vi "VP_NanoPositioner_FPGA_MultiTraj.vi"() -> ()   [LabVIEW 2015]
uses:
  FPGA states.ctl
  FPGA Commands.ctl
  RT VIs/Scan type.ctl
  Data Save Trigger.ctl
  Scan Geometry.ctl
  spiral radial direction.ctl
  spiral rotation direction.ctl
  Inner Scan axis.ctl
  Scan Type and Geometry.ctl
  Data Save Flag.ctl
  <vilib>/Platform/TimedLoop/XDataNode/timing_clust.ctl
  <vilib>/Platform/TimedLoop/XDataNode/nitl_modes.ctl
  <vilib>/Platform/TimedLoop/XDataNode/wakeup.ctl
  Trajectory FGV states.ctl
  <vilib>/rvi/Emulation/niFpgaGetClockAttributes.vi
  <vilib>/rvi/Emulation/niFpgaSctlEmulationGetInTimedLoop.vi
  <vilib>/rvi/Emulation/niFpgaEmulationReportErrorSimple.vi
  <vilib>/rvi/Emulation/niFpgaEmulationIsFPGAContextNoSignature.vi
  <vilib>/rvi/DataTransferAndStorage/Container/Common/niFpgaContainerGetUniqueNameForEmu.vi
  <vilib>/rvi/Memory/Memory_Emulation/niFpgaMemoryEmulationCacheClearOnFirstRun.vi
  <vilib>/rvi/Memory/Memory_Emulation/nirvimemoryEmulationManagerCache_MakeExclusive.vi
  <vilib>/rvi/Memory/Memory_Emulation/niFpgaMemoryEmulationValidateCache.vi
  <vilib>/rvi/Memory/Memory_Emulation/nirvimemoryEmulationManagerCache_InsertValue.vi
  <vilib>/Utility/error.llb/Clear Errors.vi
  <vilib>/rvi/Memory/Memory_Emulation/nirvimemoryEmulationManagerCache_ReleaseExclusive.vi
  <vilib>/rvi/Memory/Memory_Emulation/nirvimemoryEmulationManagerCache_GetValue.vi
  <vilib>/rvi/Memory/Memory_Emulation/nirvimemoryEmulationManagerCache_SetValue.vi
  <vilib>/rvi/Emulation/niFpgaProcessEmulError.vi
  <vilib>/rvi/Emulation/niFpgaCriticalErrorInLSC.vi
  <vilib>/rvi/interface/RandomDataEmulation/niFpgaRandomDataHandleErrors.vi
  <vilib>/rvi/eio/common/nirviEmuTemplateMethod_errors.vi
  <vilib>/rvi/DataTransferAndStorage/Container/XNode/niFpgaContainer.xnode
  <vilib>/rvi/DataTransferAndStorage/Register/Emulation/niFpgaRegisterEmulation.vi
  <vilib>/rvi/interface/RandomDataEmulation/nirviRandomDataFpgaReadWriteTemplate.vi
  <vilib>/eio/EIONode/EIONode.xnode
  <vilib>/Platform/TimedLoop/XDataNode/XDataNode.xnode
  <vilib>/Platform/TimedLoop/XDataNode/XDNodeRunTimeDep.lvlib
panel:
  in  "Data Save Flag":T1=enum."Save Data"
  out "Position Number":u32
  out "Scan Type and Geometry":T2
  out "Outer Loop iterations":i32
  out "Counter Loop iterations":i32
  in  "Y Reference DC Offset (nm)":fxp<+/-,16,16>
  in  "Y Reference Amplitude (nm)":fxp<+/-,40,17>
  in  "X Reference DC Offset (nm)":fxp<+/-,16,16>
  in  "X Reference Amplitude (nm)":fxp<+/-,40,17>
  out "Controller loop iterations":i32
  out "Trajectory Complete":bool
  in  "Inner Scan axis":T3
  in  "Spiral Rotation Direction":T4
  in  "Radial direction":T5=enum."Inward"
  in  "Det Frequency":fxp<+,32,0>=0.9999999997671694
  in  "Traj Frequency":fxp<+,32,0>=0.9999999997671694
  in  "Max radius":fxp<+/-,32,16>
  in  "Spiral Step Size":fxp<+/-,32,16>
  in  "Y Step Size":fxp<+/-,24,16>
  in  "X Step Size":fxp<+/-,24,16>
  in  "Scan Geometry":T6
  out "Z Reference Loop iterations":i32
  out "XY Reference Loop iterations":i32
  in  "Data Save Trigger Source":T7
  out "FIFO loop iterations":i32
  out "Trigger Generation Loop iterations":i32
  out "Module output loop iterations":i32
  out "Plant output loop iterations":i32
  in  "Scan type":T8
  out "Interferometer Loop Error":errorcluster
  out "Wait error":errorcluster
  out "Shutdown error":errorcluster
  out "FPGA error monitor":errorcluster
  out "Run Loop error":errorcluster
  in  "Wait timer (ms)":u16=50 caption="Count(mSec)"
  in  "New FPGA command":bool
  in  "FPGA command":T9
  out "FPGA state":T10
  out "End Run Error":errorcluster
  in  "Y End (nm)":fxp<+/-,16,16>
  in  "Y Start (nm)":fxp<+/-,16,16>
  in  "X End (nm)":fxp<+/-,16,16>
  in  "X Start (nm)":fxp<+/-,16,16>
  in  "DT Reset":bool
  in  "DT Duty Cycle (periods)":fxp<+,32,0>=0.5 caption="DT duty cycle (periods)"
  in  "DT Reference DC Offset (V)":fxp<+/-,16,16>
  in  "DT Reference Amplitude (V)":fxp<+/-,40,17>
  in  "DT Phase Offset (periods)":fxp<+,32,0>
  out "Measured Z Reference Loop Period (ticks)":u32
  in  "Z Reference Loop Period (us)":u32 caption="Z Reference Time Period (uSec)"
  in  "Z Reference DC Offset (nm)":fxp<+/-,16,16>
  in  "Z Reference Amplitude (nm)":fxp<+/-,40,17>
  in  "Detector Trigger Lower Limit (V)":fxp<+/-,20,5>=-5.0
  out "Detector Trigger In Range?":bool
  in  "Detector Trigger Upper Limit (V)":fxp<+/-,20,5>=5.0
  out "Measured Trigger Generation Loop Period (Ticks)":u32
  in  "Trigger Generation Time Period (uSec)":u32
  in  "Z-Stage Scaling Direction":fxp<+/-,3,3>=-1.0
  in  "Y-Stage Scaling Direction":fxp<+/-,3,3>=-1.0
  in  "Optics and or Sample Stage":T11(ring)
  in  "Sample Z Stage Resolution (nm)":fxp<+,33,3>=0.001000046730041504
  in  "Sample Y Stage Resolution (nm)":fxp<+,33,3>=0.001000046730041504
  in  "Sample X Stage Resolution (nm)":fxp<+,33,3>=0.001000046730041504
  out "Sample Z Stage Displacement raw (nm)":fxp<+/-,32,16> format="%.62g"
  out "Sample Y Stage Displacement raw (nm)":fxp<+/-,32,16> format="%.41g"
  out "Sample X Stage Displacement raw (nm)":fxp<+/-,32,16> format="%.62g"
  in  "Reset Sample Z":bool
  in  "Reset Sample Y":bool
  in  "Reset Sample X":bool
  out "Mod6/DIO3":bool
  out "Mod6/DIO2":bool
  out "Mod5/DIO3":bool
  out "Mod5/DIO2":bool
  out "Mod4/DIO3":bool
  out "Mod4/DIO2":bool
  in  "X-Stage Scaling Direction":fxp<+/-,3,3>=-1.0
  in  "Z-Stage nm to V Scaling":fxp<+/-,32,12>
  in  "Y-Stage nm to V Scaling":fxp<+/-,32,12>
  in  "X-Stage nm to V Scaling":fxp<+/-,32,12>
  out "Kxx Output, Kxx*ex (V)":fxp<+/-,58,25>
  out "Kyy Output, Kyy*ey (V)":fxp<+/-,58,25>
  out "Kzz Output, Kzz*ez (V)":fxp<+/-,58,25>
  in  "sos gain SF Controller xx1":fxp<+/-,42,9>
  in  "-a01(2) xx1":fxp<+/-,64,9>[](array[numeric])=[0.0, 0.0, 0.0, 0.0, 0.0, 0.0, 0.0, 0.0, 0.0, 0.0, 0.0, 0.0, 0.0, 0.0, 0.0, 0.0, 0.0, 0.0, 0.0, 0.0]
  in  "-a02(2) xx1":fxp<+/-,64,9>[](array[numeric])=[0.0, 0.0, 0.0, 0.0, 0.0, 0.0, 0.0, 0.0, 0.0, 0.0, 0.0, 0.0, 0.0, 0.0, 0.0, 0.0, 0.0, 0.0, 0.0, 0.0]
  in  "b01(2) xx1":fxp<+/-,64,9>[](array[numeric])=[0.0, 0.0, 0.0, 0.0, 0.0, 0.0, 0.0, 0.0, 0.0, 0.0, 0.0, 0.0, 0.0, 0.0, 0.0, 0.0, 0.0, 0.0, 0.0, 0.0]
  in  "b02(2) xx1":fxp<+/-,64,9>[](array[numeric])=[0.0, 0.0, 0.0, 0.0, 0.0, 0.0, 0.0, 0.0, 0.0, 0.0, 0.0, 0.0, 0.0, 0.0, 0.0, 0.0, 0.0, 0.0, 0.0, 0.0]
  in  "sos gain SF Controller yy1":fxp<+/-,42,9>
  in  "-a01(2) yy1":fxp<+/-,64,9>[](array[numeric])=[0.0, 0.0, 0.0, 0.0, 0.0, 0.0, 0.0, 0.0, 0.0, 0.0, 0.0, 0.0, 0.0, 0.0, 0.0, 0.0, 0.0, 0.0, 0.0, 0.0]
  in  "-a02(2) yy1":fxp<+/-,64,9>[](array[numeric])=[0.0, 0.0, 0.0, 0.0, 0.0, 0.0, 0.0, 0.0, 0.0, 0.0, 0.0, 0.0, 0.0, 0.0, 0.0, 0.0, 0.0, 0.0, 0.0, 0.0]
  in  "b01(2) yy1":fxp<+/-,64,9>[](array[numeric])=[0.0, 0.0, 0.0, 0.0, 0.0, 0.0, 0.0, 0.0, 0.0, 0.0, 0.0, 0.0, 0.0, 0.0, 0.0, 0.0, 0.0, 0.0, 0.0, 0.0]
  in  "b02(2) yy1":fxp<+/-,64,9>[](array[numeric])=[0.0, 0.0, 0.0, 0.0, 0.0, 0.0, 0.0, 0.0, 0.0, 0.0, 0.0, 0.0, 0.0, 0.0, 0.0, 0.0, 0.0, 0.0, 0.0, 0.0]
  in  "sos gain SF Controller zz1":fxp<+/-,42,9>
  in  "-a01(2) zz1":fxp<+/-,64,9>[](array[numeric])=[0.0, 0.0, 0.0, 0.0, 0.0, 0.0, 0.0, 0.0, 0.0, 0.0, 0.0, 0.0, 0.0, 0.0, 0.0, 0.0, 0.0, 0.0, 0.0, 0.0]
  in  "-a02(2) zz1":fxp<+/-,64,9>[](array[numeric])=[0.0, 0.0, 0.0, 0.0, 0.0, 0.0, 0.0, 0.0, 0.0, 0.0, 0.0, 0.0, 0.0, 0.0, 0.0, 0.0, 0.0, 0.0, 0.0, 0.0]
  in  "b01(2) zz1":fxp<+/-,64,9>[](array[numeric])=[0.0, 0.0, 0.0, 0.0, 0.0, 0.0, 0.0, 0.0, 0.0, 0.0, 0.0, 0.0, 0.0, 0.0, 0.0, 0.0, 0.0, 0.0, 0.0, 0.0]
  in  "b02(2) zz1":fxp<+/-,64,9>[](array[numeric])=[0.0, 0.0, 0.0, 0.0, 0.0, 0.0, 0.0, 0.0, 0.0, 0.0, 0.0, 0.0, 0.0, 0.0, 0.0, 0.0, 0.0, 0.0, 0.0, 0.0]
  in  "Scaling mV to V":fxp<+,33,10>=0.0009765625
  in  "System Loop Type":enum16{"Open Loop", "Closed Loop"}(ring)
  in  "Timeout FPGA FIFO1":i32=40000000
  out "FIFO Timed Out":bool
  out "Number of Data Strings":i32
  out "Optics Z Stage Displacement raw (nm)":fxp<+/-,32,16>
  in  "Optics Z Stage Resolution (nm)":fxp<+,33,3>=0.001000046730041504
  in  "Reset Optics Z":bool
  out "Mod6/DIO1":bool
  out "Mod6/DIO0":bool
  out "Optics Y Stage Displacement raw (nm)":fxp<+/-,32,16>
  in  "Optics Y Stage Resolution (nm)":fxp<+,33,3>=0.001000046730041504
  in  "Reset Optics Y":bool
  out "Mod5/DIO1":bool
  out "Mod5/DIO0":bool
  out "Z-Stage Input In Range?":bool
  out "Y-Stage Input In Range?":bool
  in  "Controller Output Lower Limit":fxp<+/-,20,5>=-5.0
  out "X-Stage Input In Range?":bool
  in  "Controller Output Upper Limit":fxp<+/-,20,5>=5.0
  out "Measured Counter Time Period (Ticks)":u32
  out "Measured Datalog Period (Ticks)":u32
  out "Measured Plant Output Loop Period (Ticks)":u32
  out "Measured Module Output Loop Period (Ticks)":u32
  out "Measured Controller Loop Period (Ticks)":u32
  out "Measured XY Reference Loop Period (ticks)":u32
  out "Optics X Stage Displacement raw (nm)":fxp<+/-,32,16>
  in  "Optics X Stage Resolution (nm)":fxp<+,33,3>=0.001000046730041504 format="%#_31g"
  in  "Plant Output Loop Period (uSec)":u32 caption="Plant Output Time Period (uSec)"
  in  "Reset Optics X":bool
  out "Mod4/DIO1":bool
  out "Mod4/DIO0":bool
  out "Start Run Error":errorcluster
  out "Stop Scan":bool
  in  "Module Output Loop Period (uSec)":u32 caption="Controller Output Time Period (uSec)"
  in  "Datalog Cases":T12(ring)
  in  "Controller Loop Period (uSec)":u32 caption="Controller Time Period (uSec)"
  in  "FIFO Loop Period (us)":u32 caption="Datalog Time Period (uSec)"
  in  "XY Reference Loop Period (us)":u32 caption="X Reference Time Period (uSec)"
  out "FIFO Timed Out?":bool
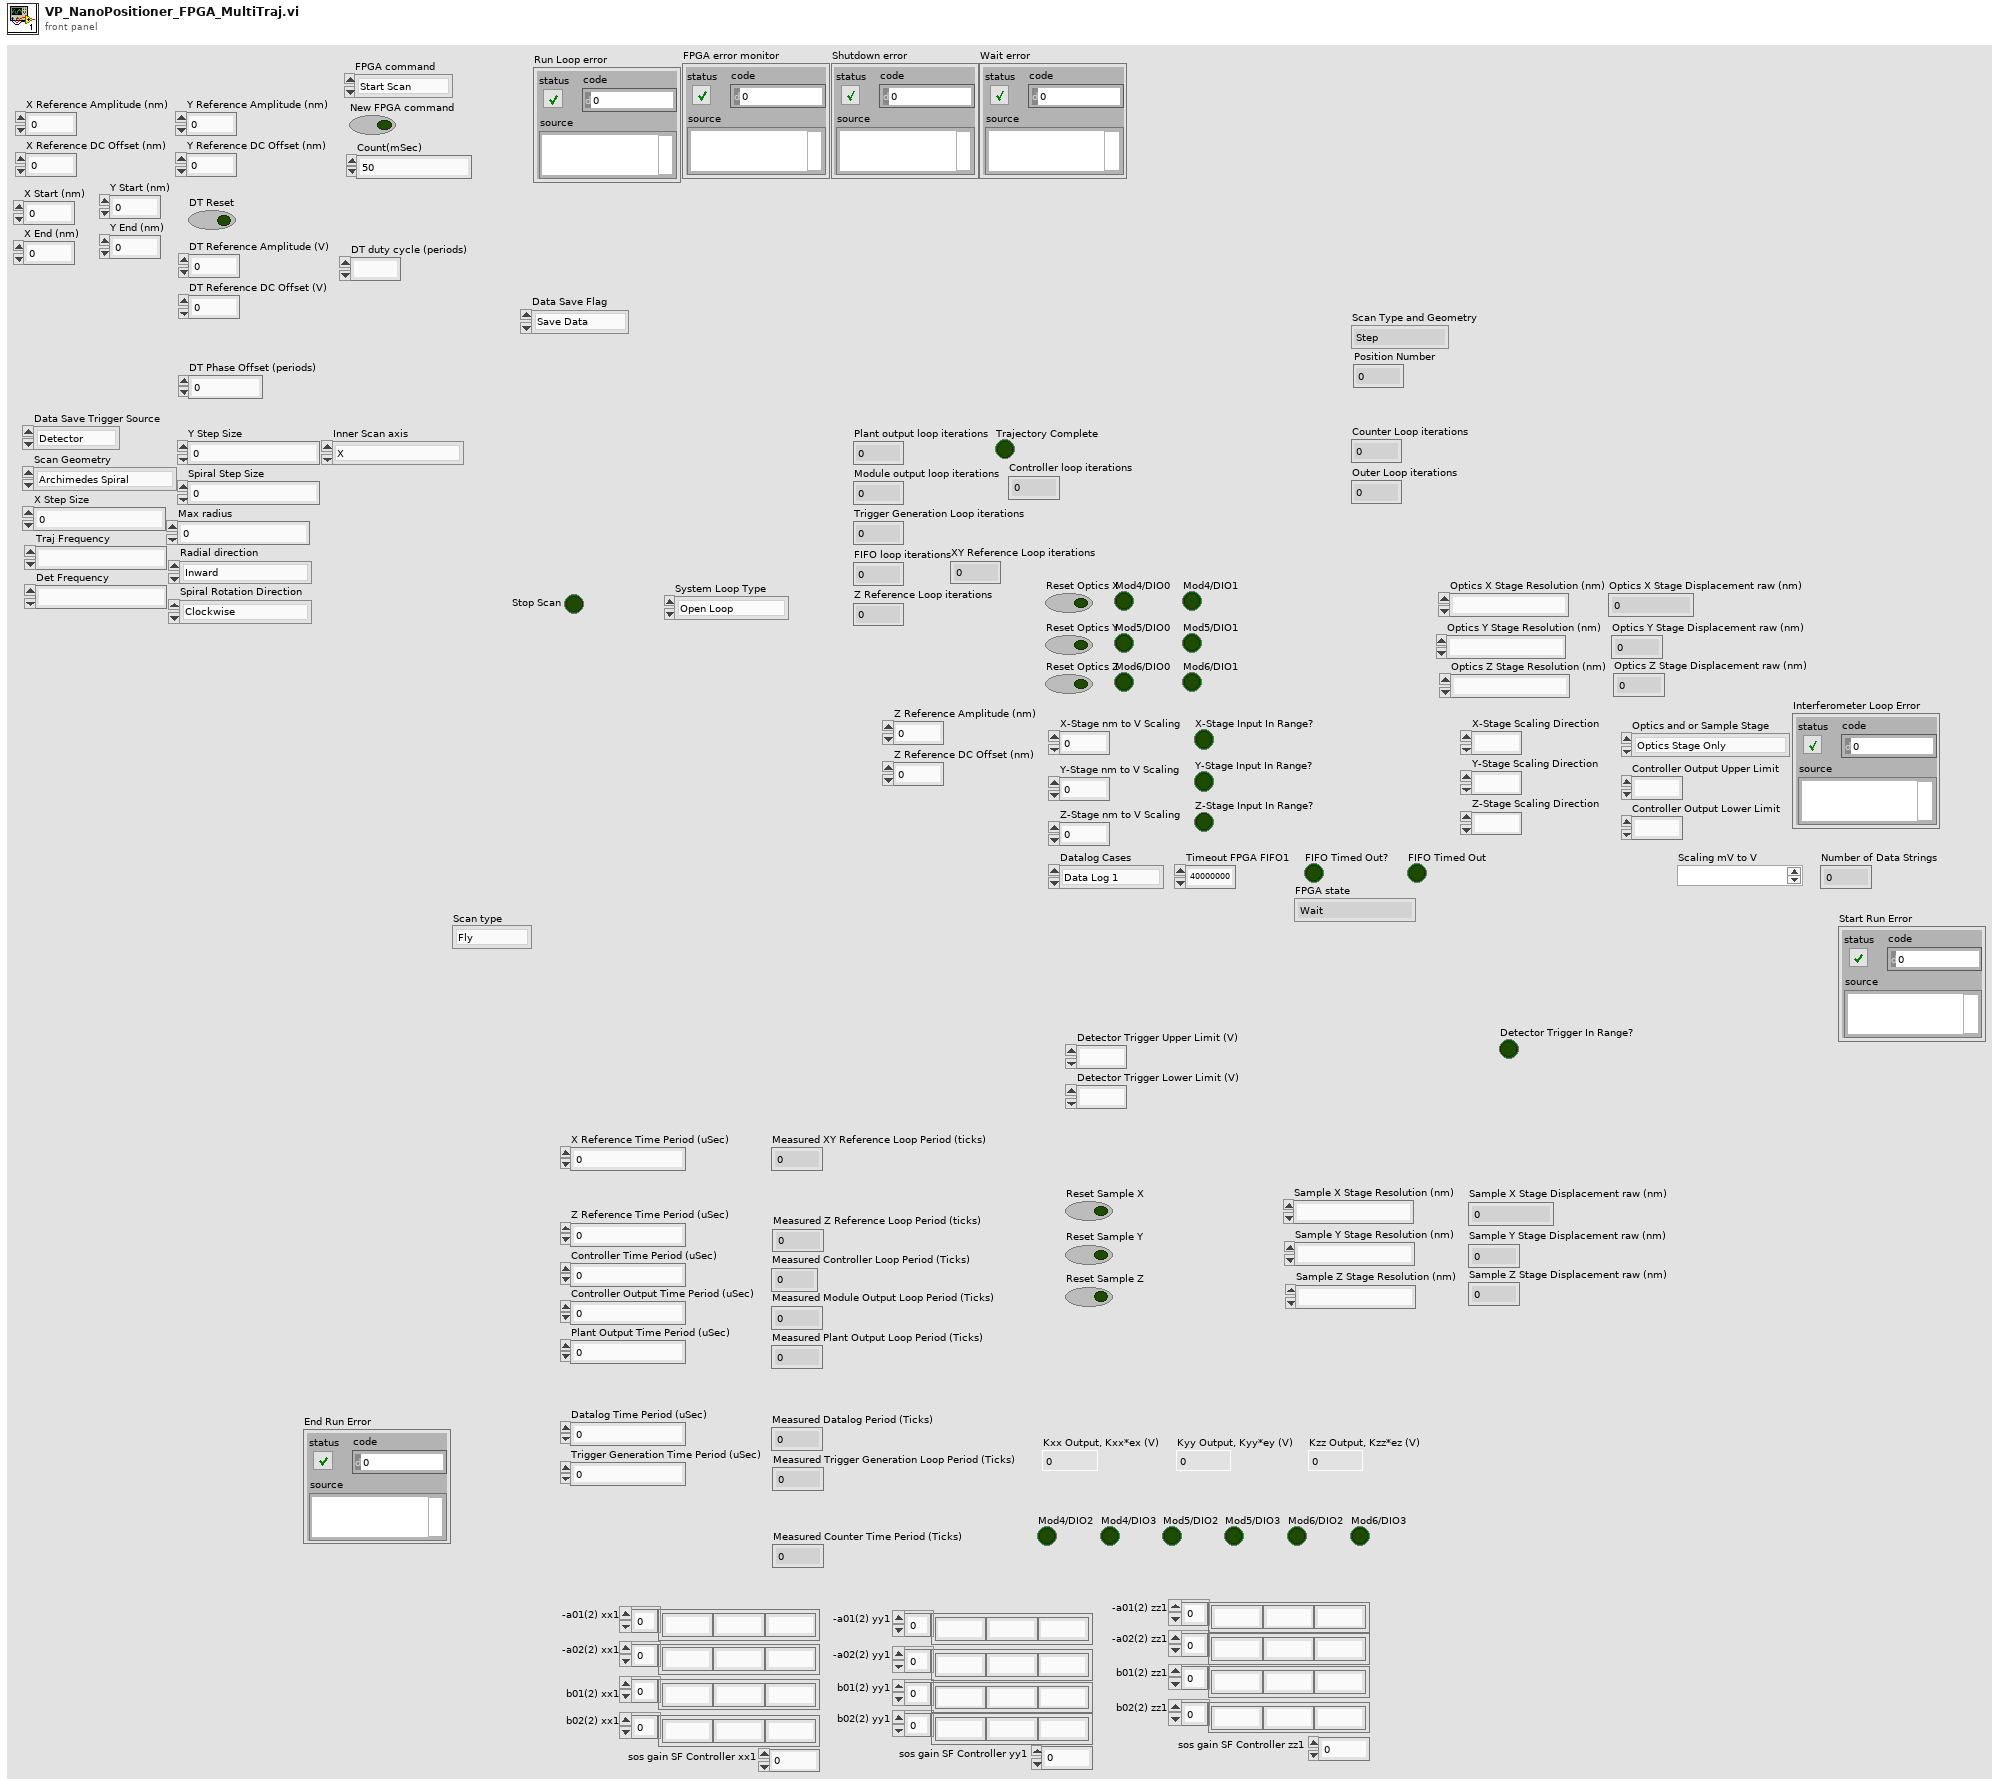
[diagram p1: front panel]
types:
  T1 = typedef "Data Save Flag.ctl" = enum16{"Skip Data", "Save Data"}
  T2 = typedef "Scan Type and Geometry.ctl" = enum16{"Step", "Fly Arch Spiral", "Fly Snake", "Fly Grid Spiral"}
  T3 = typedef "Inner Scan axis.ctl" = enum16{"X", "Y"}
  T4 = typedef "spiral rotation direction.ctl" = enum16{"Clockwise", "Anti-clockwise"}
  T5 = typedef "spiral radial direction.ctl" = enum16{"Outward", "Inward"}
  T6 = typedef "Scan Geometry.ctl" = enum16{"Archimedes Spiral", "Grid Spiral", "Snake"}
  T7 = typedef "Data Save Trigger.ctl" = enum16{"Detector", "Trajectory"}
  T8 = typedef "Scan type.ctl" = enum16{"Fly", "Step"}
  T9 = typedef "FPGA Commands.ctl" = enum16{"Start Scan", "Shutdown"}
  T10 = typedef "FPGA states.ctl" = enum16{"Wait", "Start Run", "Run", "End Run", "Shutdown"}
  T11 = enum16{"Optics Stage Only", "Optics and Sample Stage"}
  T12 = enum16{"Data Log 1", "Data Log 2", "Data Log 3", "Data Log 4", "Data Log 5", "Data Log 6", "Data Log 7", "Data Log 8", "Data Log 9", "Data Log 10", "Data Log 11", "Data Log 12", "Data Log 13", "Data Log 14", "Data Log 15", "Data Log 16"}
  T13 = typedef "Trajectory FGV states.ctl" = enum16{"Initialize", "Increment"}
  T14 = typedef "XDNodeRunTimeDep.lvlib/timing_clust.ctl" = cluster{"Expected End [f-1]":u64, "Actual End [f-1]":u64, "Finished Late? [f-1]":bool, "Expected End [i-1]":u64, "Actual End [i-1]":u64, "Finished Late? [i-1]":bool, "Expected Start [i]":u64, "Actual Start [i]":u64, "Expected Start [f]":u64, "Actual Start [f]":u64, "Source Name":string, "Structure Name":string, "Period":i64, "Deadline":i64, "Offset":i64, "Start":i64, "Priority":i32, "Timeout":i32, "Mode":T15, "Wakeup Reason":T16, "Error":errorcluster, "Source Type":string, "Secondary Source Type":string, "Global End Time":u64, "Global Start Time":u64, "Frame Duration":u64, "Iteration Duration":u64, "Assigned CPU":i32, "I/O Scan Engine Mode":u32}
  T15 = typedef "XDNodeRunTimeDep.lvlib/nitl_modes.ctl" = enum32{"No Change", "Process missed periods, maintain original phase", "Discard missed periods, maintain original phase", "Process missed periods, ignore original phase", "Discard missed periods, ignore original phase"}
  T16 = typedef "XDNodeRunTimeDep.lvlib/wakeup.ctl" = enum32{"Normal", "Aborted", "Asynchronous wakeup", "Timing source error", "Timed loop error", "Timeout"}
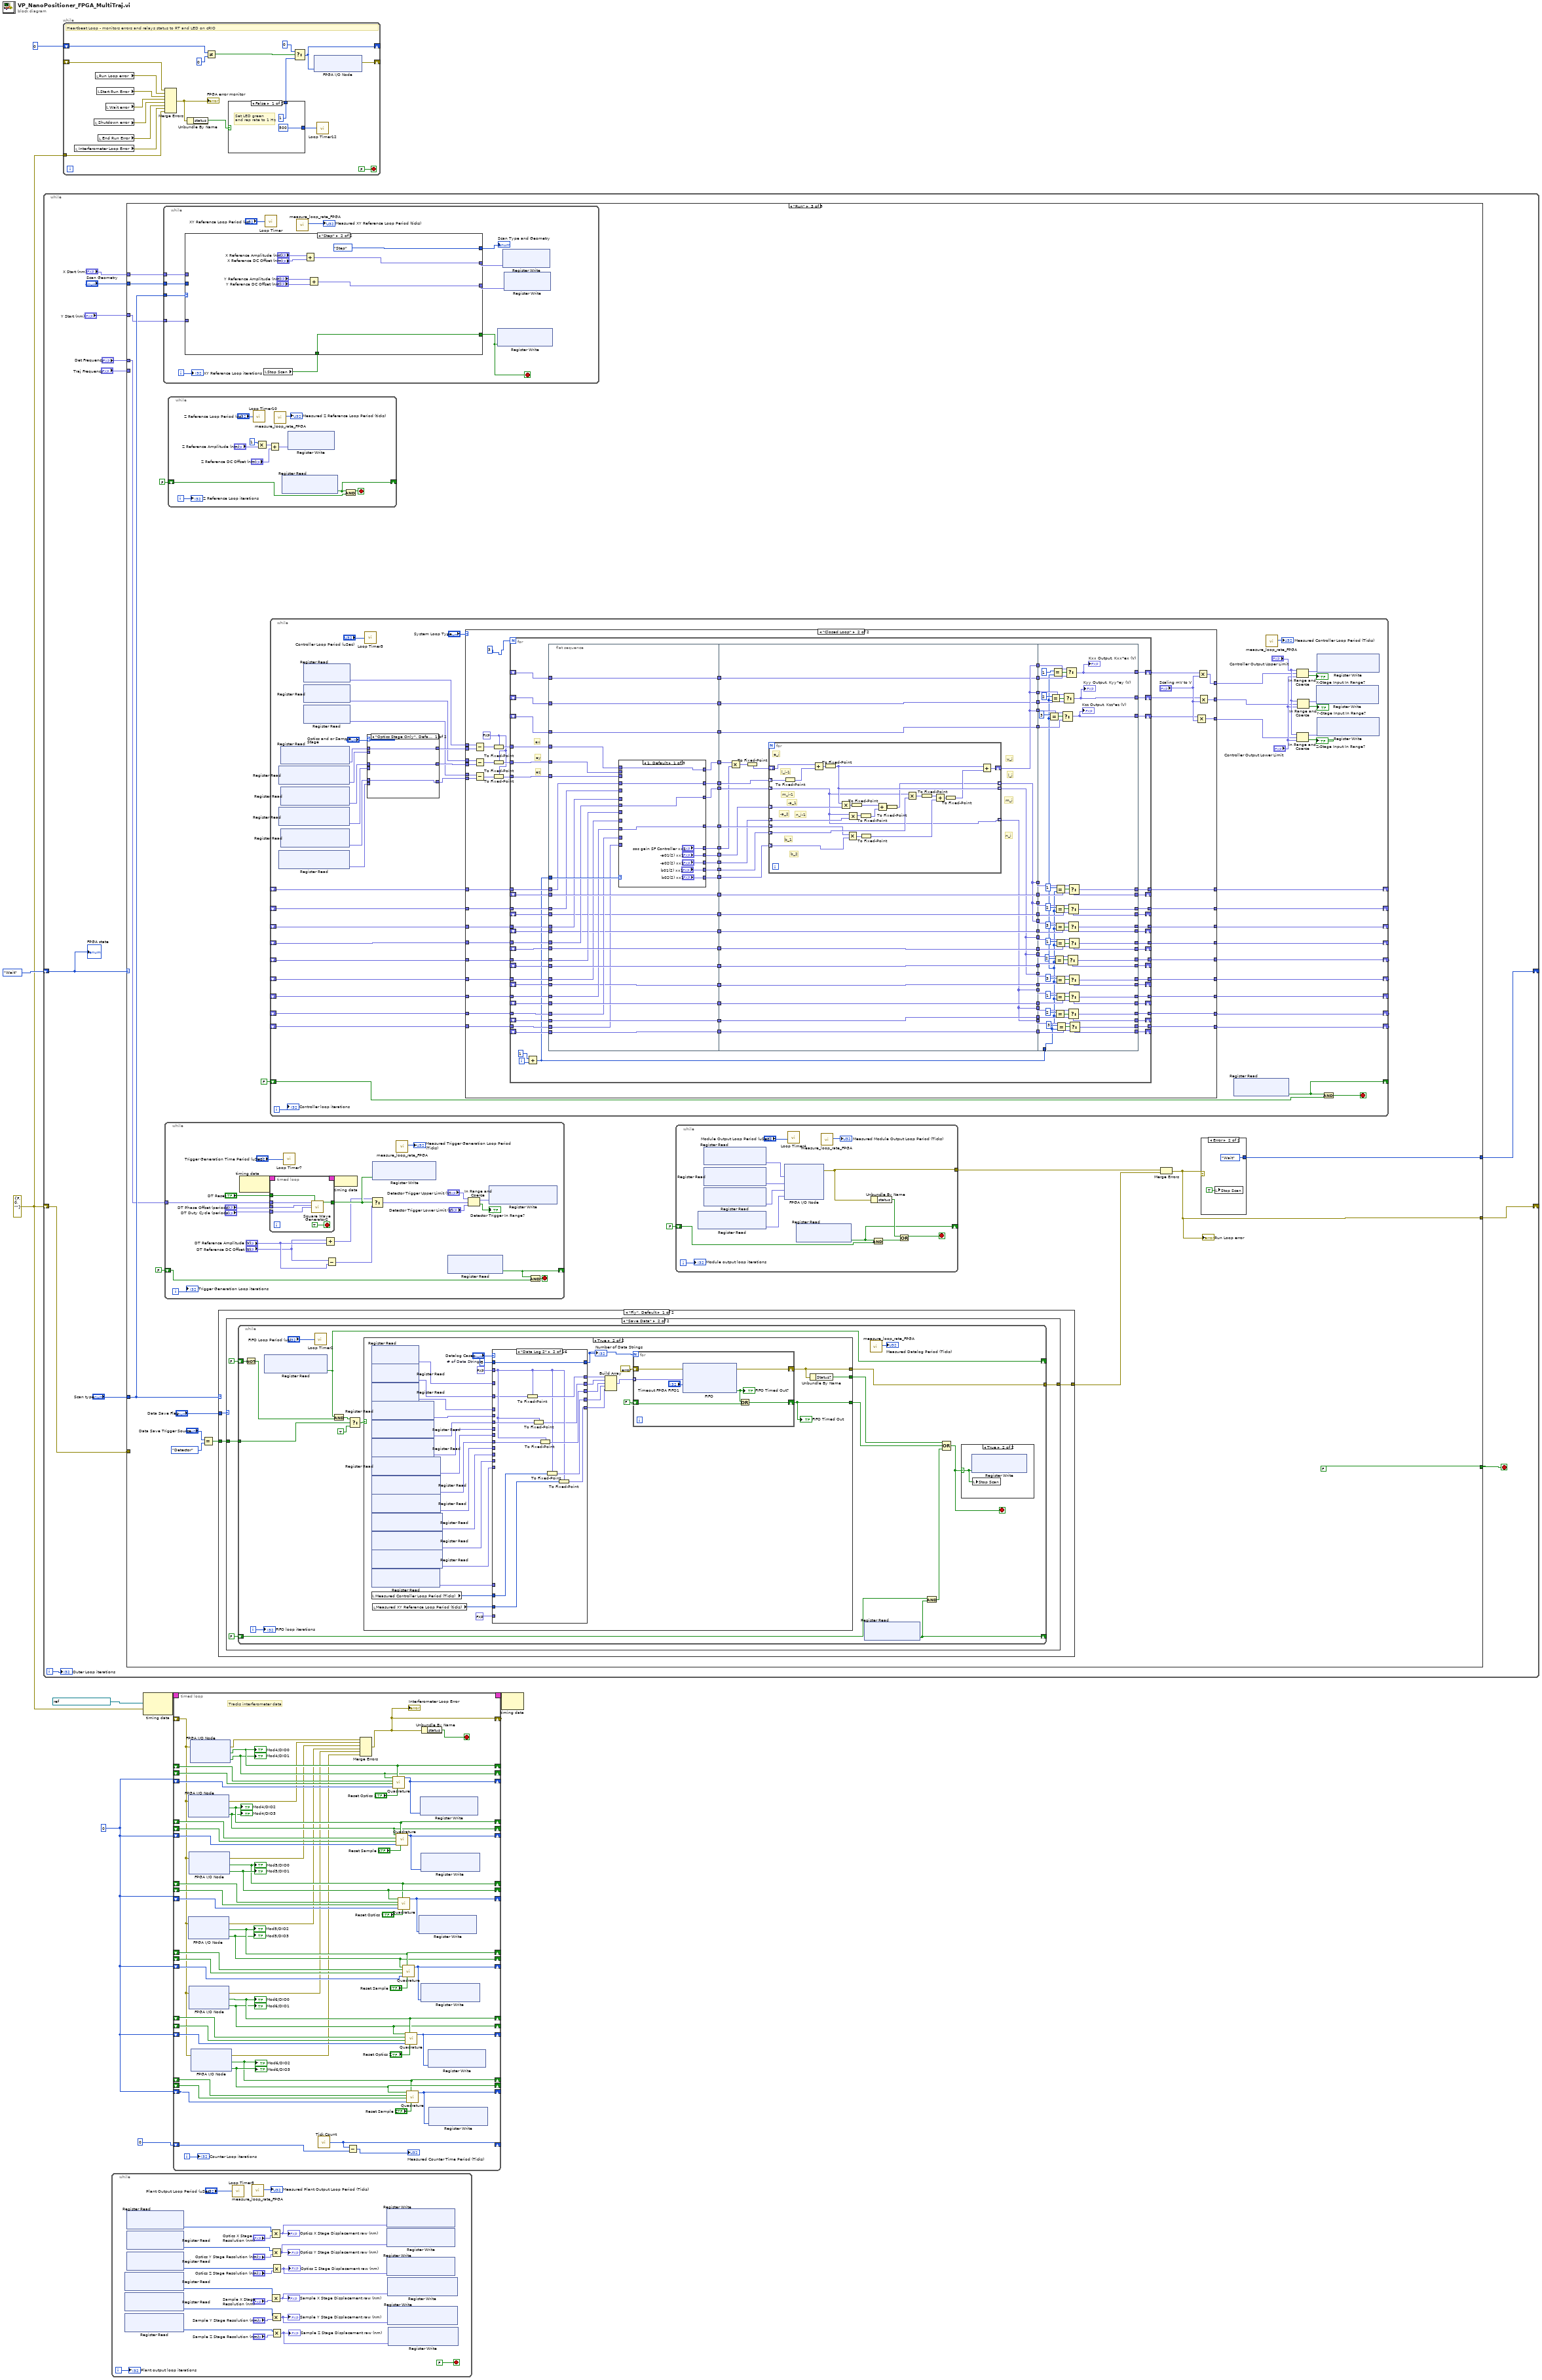
[diagram p0: block diagram]
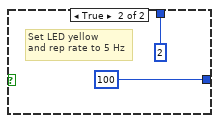
[diagram p2: hidden frame]
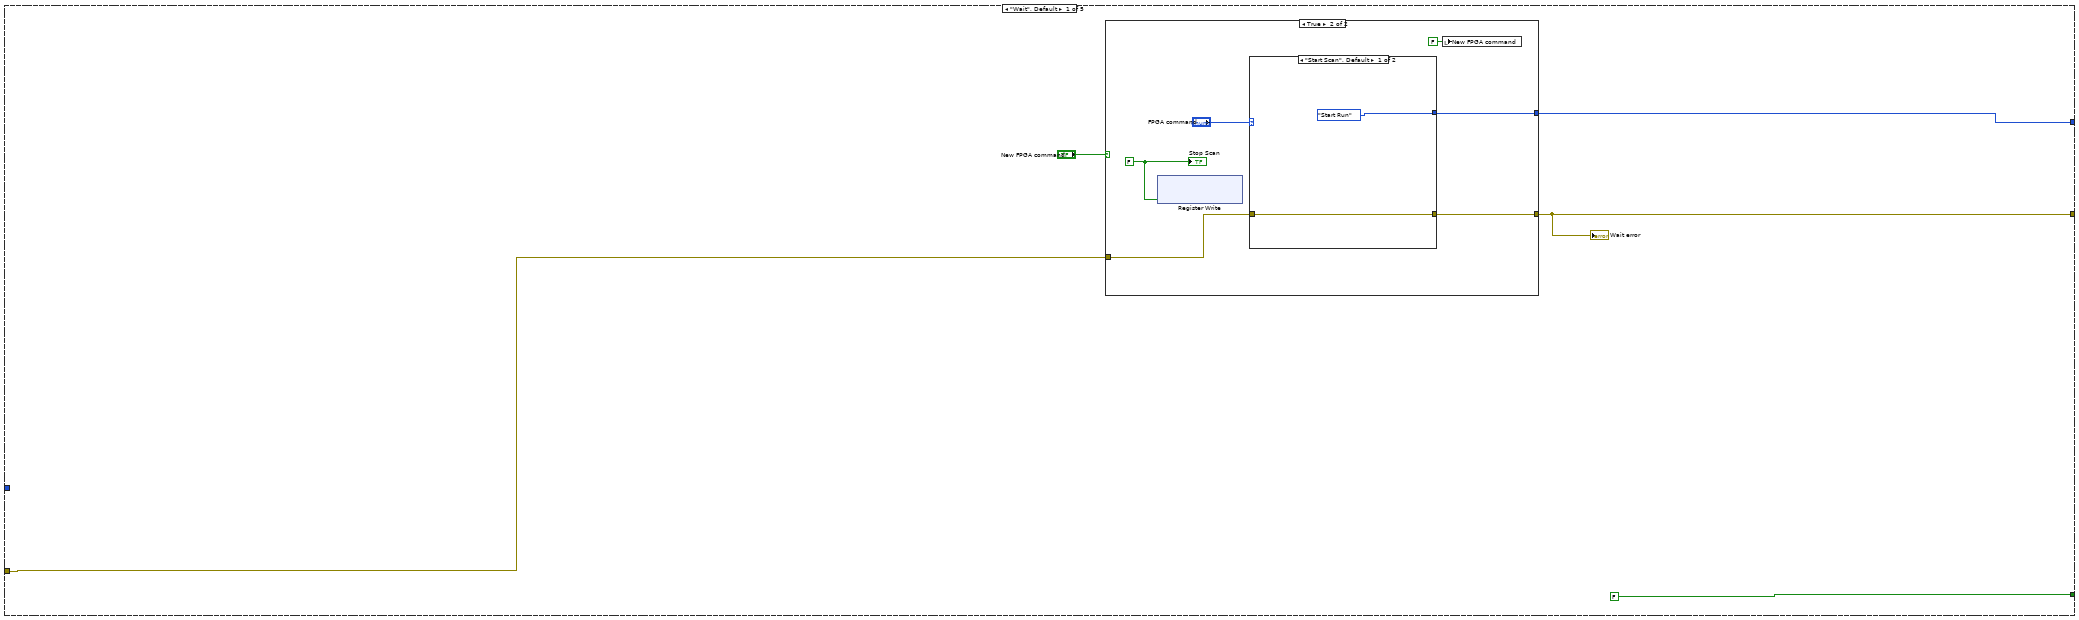
[diagram p3: hidden frame]
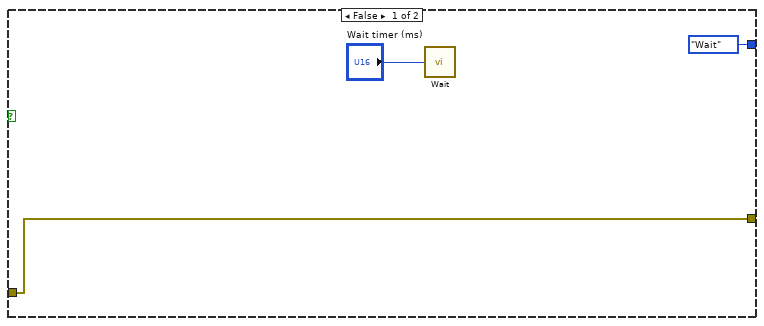
[diagram p4: hidden frame]
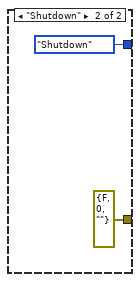
[diagram p5: hidden frame]
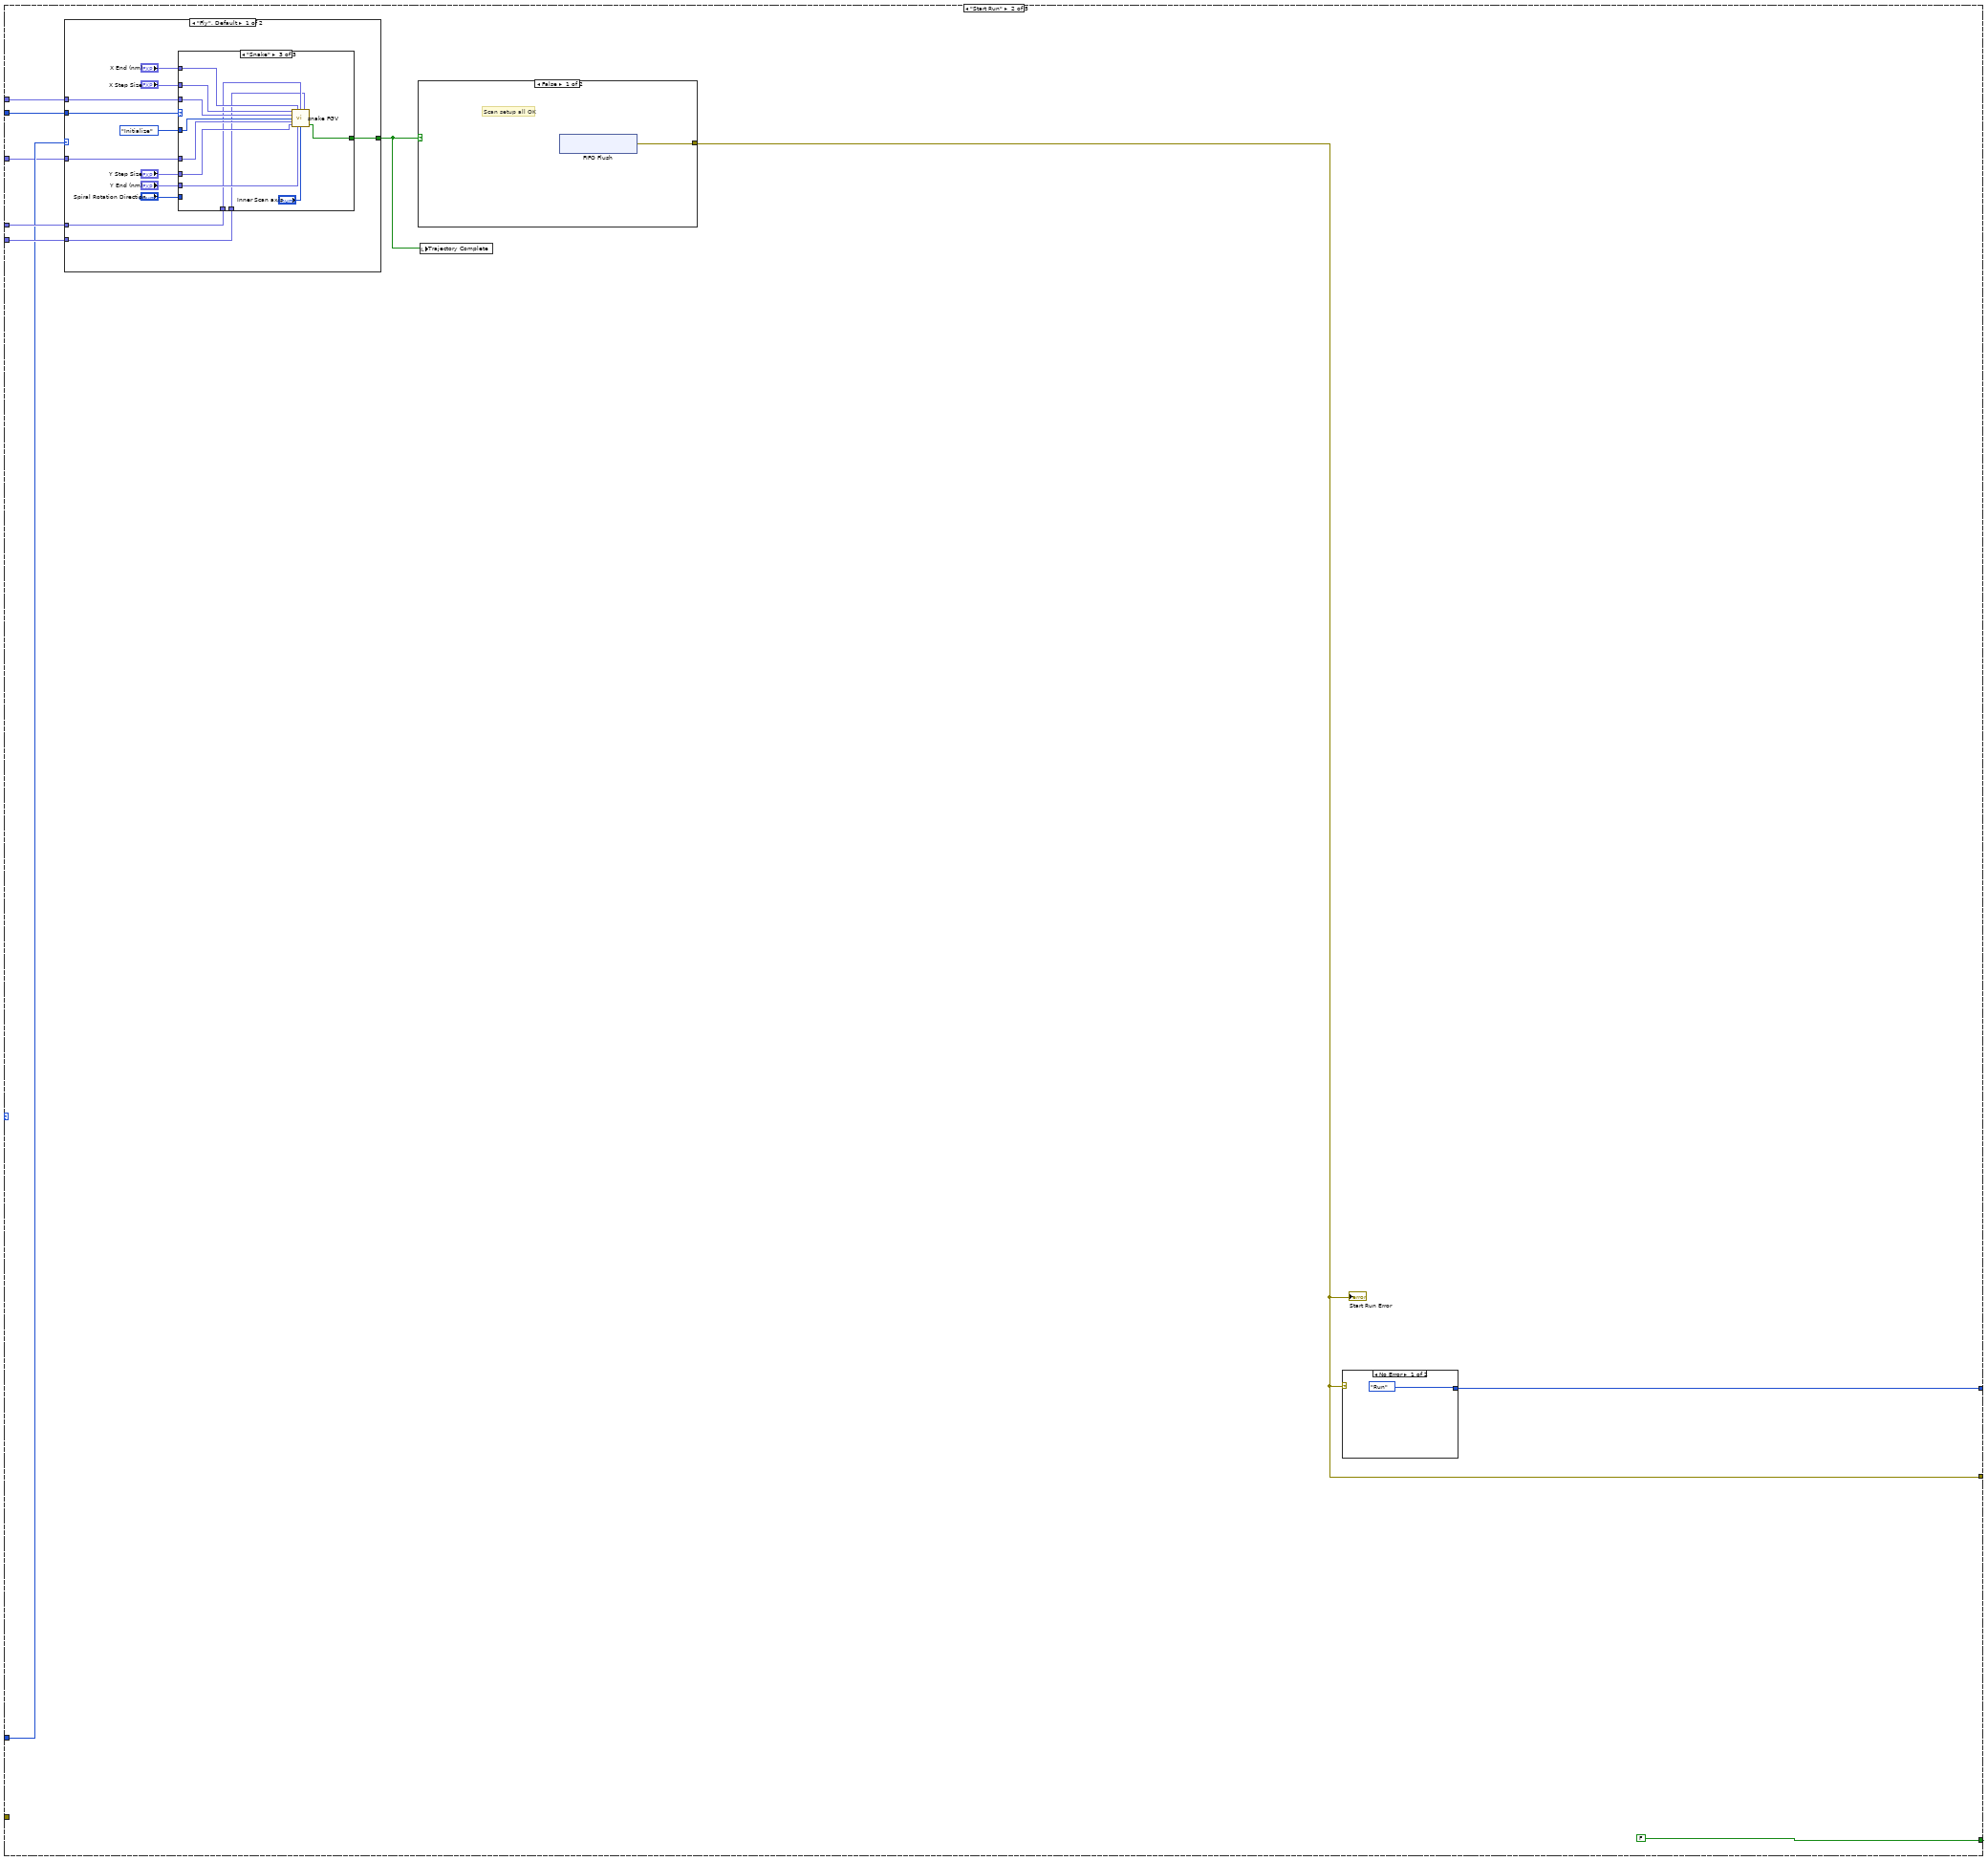
[diagram p6: hidden frame]
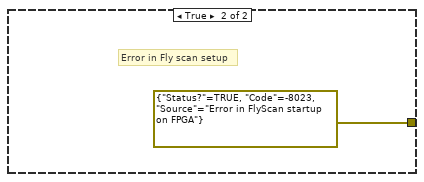
[diagram p7: hidden frame]
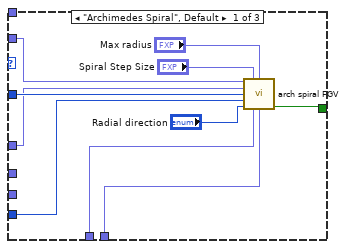
[diagram p8: hidden frame]
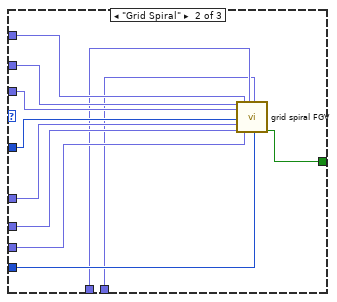
[diagram p9: hidden frame]
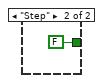
[diagram p10: hidden frame]
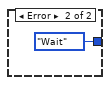
[diagram p11: hidden frame]
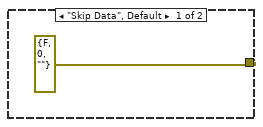
[diagram p12: hidden frame]
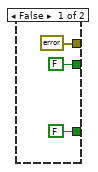
[diagram p13: hidden frame]
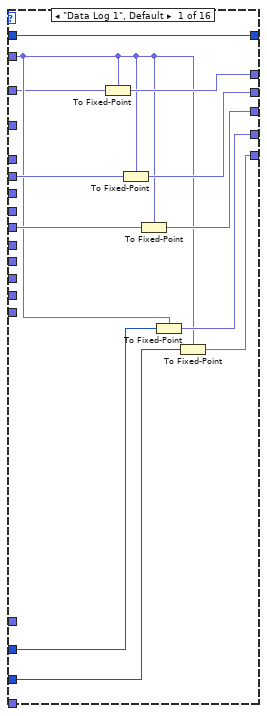
[diagram p14: hidden frame]
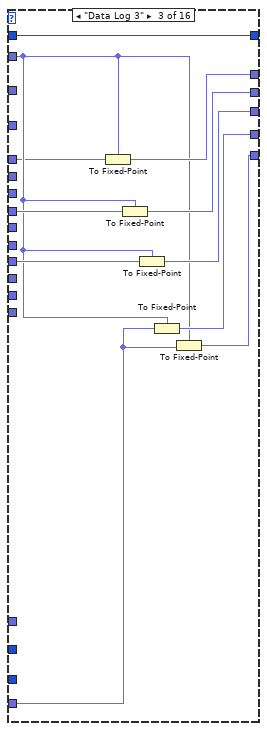
[diagram p15: hidden frame]
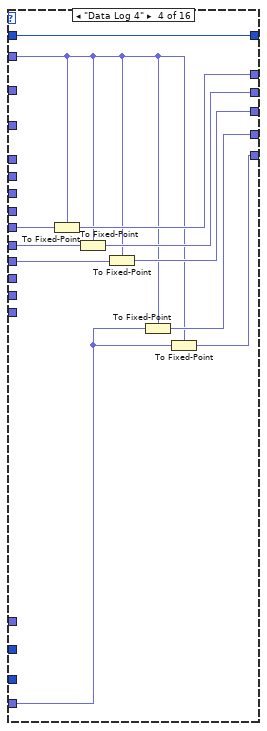
[diagram p16: hidden frame]
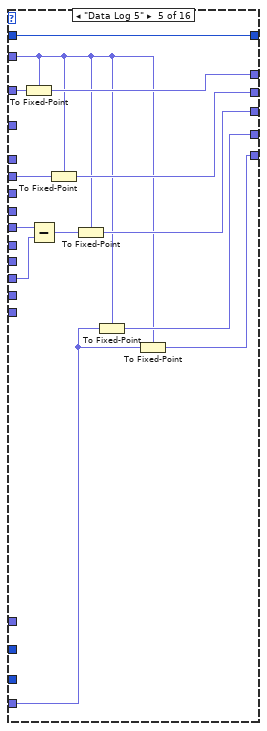
[diagram p17: hidden frame]
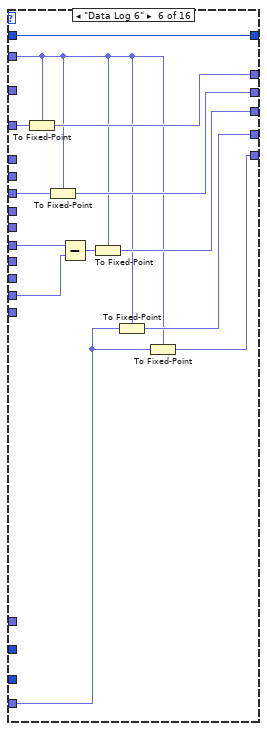
[diagram p18: hidden frame]
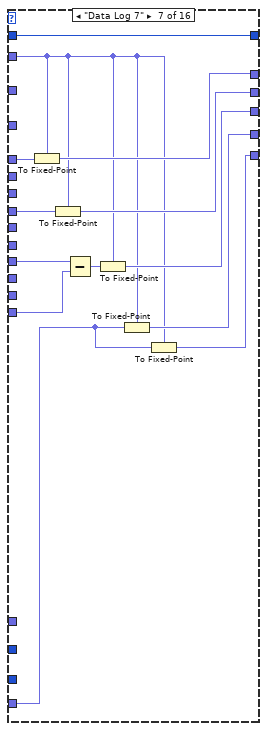
[diagram p19: hidden frame]
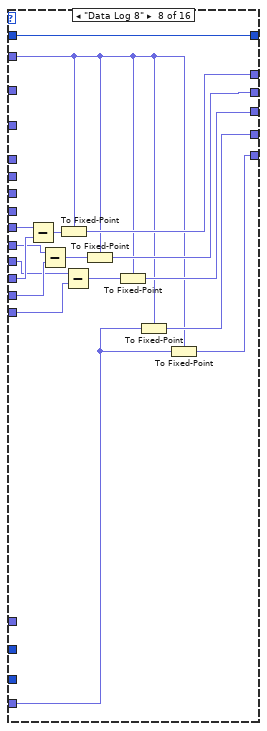
[diagram p20: hidden frame]
diagram:
  w4 = 0 ("Tick Count(Ticks)")
  w1 = errorcluster {"status"=FALSE, "code"=0, "source"=""} ("error IO")
  n1 = while {
    shift-right: [w12] -> _
    shift-left: FPGA_states."Wait" -> [w20]
    shift-right: [w17] -> _
    shift-left: w1 -> [w18]
    i -> [w11]
    stop <- w19 stop-if-true
    n2 = case shown="\"Run\"" w20 {
      tunnel: [w24 w42 w112 w870 w877] -> w17
      tunnel: [FALSE FALSE FALSE FALSE TRUE] -> w19
      tunnel: [w21 w43 w113 FPGA_states."Wait" FPGA_states."Shutdown"] -> w12
      tunnel: w18 -> [w22 _ _ w871 w878]
      tunnel: "Scan Geometry" -> [_ w47 w109 _ _]
      tunnel: "Traj Frequency" -> [_ w46 _ _ _]
      tunnel: "Det Frequency" -> [_ w45 w104 _ _]
      tunnel: "Scan type" -> [_ w44 w105 _ _]
      tunnel: "X Start (nm)" -> [_ w40 w99 _ _]
      tunnel: "Y Start (nm)" -> [_ w39 w100 _ _]
      frame "Wait", Default {
        n3 = case shown="True" "New FPGA command" {
          tunnel: [FPGA_states."Wait" w34] -> w21
          tunnel: w22 -> [w28 w33]
          tunnel: [w28 w32] -> w24
          frame False {
            n4 = call "Wait"("Count(mSec)"="Wait timer (ms)") -> ()  [unwired: 1 out]
          }
          frame True {
            w29 = FALSE ("stop case")
            n5 = xnode ("Register Write")("Data"=w29) -> ()  [unwired: 1 in, 1 out]
            n6 = case shown="\"Start Scan\", Default" "FPGA command" {
              tunnel: [FPGA_states."Start Run" FPGA_states."Shutdown"] -> w34
              tunnel: w33 -> [w35 _]
              tunnel: [w35 errorcluster {"status"=FALSE, "code"=0, "source"=""} ("error IO")] -> w32
              frame "Start Scan", Default {
              }
              frame "Shutdown" {
              }
            }
            n7 = local write "New FPGA command"(FALSE ("New FPGA command")) -> ()
            "Stop Scan" <- w29
          }
        }
        "Wait error" <- w24
      }
      frame "Start Run" {
        n8 = case shown="\"Fly\", Default" w44 {
          tunnel: w47 -> [w61 _]
          tunnel: w46 -> [w60 _]
          tunnel: w45 -> [w59 _]
          tunnel: [w53 FALSE ("Trajectory Complete")] -> w41
          tunnel: w40 -> [w52 _]
          tunnel: w39 -> [w51 _]
          frame "Fly", Default {
            n9 = case shown="\"Snake\"" w61 {
              tunnel: Trajectory_FGV_states."Initialize" ("Action") -> [w72 w83 w94]
              tunnel: [w71 w82 w93] -> w53
              tunnel: w52 -> [w70 w81 w92]
              tunnel: "X Step Size" -> [_ w80 w91]
              tunnel: "X End (nm)" -> [_ w79 w90]
              tunnel: w51 -> [w69 w78 w89]
              tunnel: "Y Step Size" -> [_ w77 w88]
              tunnel: "Y End (nm)" -> [_ w76 w87]
              tunnel: w60 -> [w66 w73 w85]
              tunnel: w59 -> [w65 w74 w86]
              tunnel: "Spiral Rotation Direction" -> [w63 w75 _]
              frame "Archimedes Spiral", Default {
                n10 = call "arch spiral FGV.vi"("X Start"=w70, "Spiral Step Size"="Spiral Step Size", "Max radius"="Max radius", "Y Start"=w69, "Action"=w72, "Spiral Rotation Direction"=w63, "Radial direction"="Radial direction", "Det Frequency"=w65, "Traj Frequency"=w66) -> ("Trajectory Complete"=w71:bool)  [unwired: 3 in, 3 out]
              }
              frame "Grid Spiral" {
                n11 = call "grid spiral FGV.vi"("X Step Size"=w80, "X Start"=w81, "Action"=w83, "Y Start"=w78, "Y Step Size"=w77, "X End"=w79, "Y End"=w76, "Det Frequency"=w74, "Traj Frequency"=w73, "Spiral Rotation Direction"=w75) -> ("Trajectory Complete"=w82:bool)  [unwired: 2 in, 7 out]
              }
              frame "Snake" {
                n12 = call "snake FGV.vi"("X Step Size"=w91, "X End"=w90, "Det Frequency"=w86, "Traj Frequency"=w85, "X Start"=w92, "Action"=w94, "Y Start"=w89, "Y Step Size"=w88, "Y End"=w87, "Inner Scan axis"="Inner Scan axis") -> ("Trajectory Complete"=w93:bool)  [unwired: 2 in, 3 out]
              }
            }
          }
          frame "Step" {
          }
        }
        n13 = case shown="False" w41 {
          tunnel: [w49 errorcluster {"Status?"=TRUE, "Code"=-8023, "Source"="Error in FlyScan startup on FPGA"} ("error out")] -> w42
          frame False {
            # "Scan setup all OK"
            n14 = xnode ("FIFO Flush")() -> ("error out"=w49:errorcluster)  [unwired: 2 in, 1 out]
          }
          frame True {
            # "Error in Fly scan setup"
          }
        }
        "Start Run Error" <- w42
        n15 = local write "Trajectory Complete"(w41) -> ()
        n16 = case shown="No Error" w42 {
          tunnel: [FPGA_states."Run" FPGA_states."Wait"] -> w43
          frame No Error {
          }
          frame Error {
          }
        }
      }
      frame "Run" {
        n17 = while {
          tunnel: w109 -> [w823]
          tunnel: w105 -> [w818]
          tunnel: w100 -> [w816]
          tunnel: w99 -> [w815]
          i -> [w824]
          stop <- w819 stop-if-true
          n18 = local read "Stop Scan"() -> (w820:bool)
          n19 = case shown="\"Step\"" w818 {
            tunnel: w823 -> [w839 _]
            tunnel: [w832 w866] -> w822
            tunnel: [w830 w863] -> w821
            tunnel: w820 -> [w836 w869]
            tunnel: [w835 w869] -> w819
            tunnel: [w834 Scan_Type_and_Geometry."Step"] -> w817
            tunnel: w816 -> [w828 _]
            tunnel: w815 -> [w827 _]
            frame "Fly", Default {
              n20 = case shown="\"Archimedes Spiral\", Default" w839 {
                tunnel: Trajectory_FGV_states."Increment" ("Action") -> [w849 w855 w861]
                tunnel: [w848 w854 w860] -> w829
                tunnel: [w847 w853 w859] -> w833
                tunnel: [w846 w852 w858] -> w831
                tunnel: [w845 w851 w857] -> w837
                tunnel: [Scan_Type_and_Geometry."Fly Arch Spiral" Scan_Type_and_Geometry."Fly Grid Spiral" Scan_Type_and_Geometry."Fly Snake"] -> w834
                frame "Archimedes Spiral", Default {
                  n21 = call "arch spiral FGV.vi"("Action"=w849) -> ("X position"=w847:fxp<+/-,32,16>, "Y position"=w846:fxp<+/-,32,16>, "Number of positions"=w845:u32, "Trajectory Complete"=w848:bool)  [unwired: 11 in]
                }
                frame "Grid Spiral" {
                  n22 = call "grid spiral FGV.vi"("Action"=w855) -> ("X position"=w853:fxp<+/-,32,16>, "Y position"=w852:fxp<+/-,32,16>, "Number of positions"=w851:u32, "Trajectory Complete"=w854:bool)  [unwired: 11 in, 4 out]
                }
                frame "Snake" {
                  n23 = call "snake FGV.vi"("Action"=w861) -> ("X position"=w859:fxp<+/-,32,16>, "Y position"=w858:fxp<+/-,32,16>, "Number of positions"=w857:u32, "Trajectory Complete"=w860:bool)  [unwired: 11 in]
                }
              }
              "Trajectory Complete" <- w829
              "Position Number" <- w837
              n24 = xnode ("Register Write")("Data"=w837) -> ()  [unwired: 1 in, 1 out]
              n25 = Or(x=w829, y=w836) -> (x .or. y?=w835:bool)
              n26 = case shown="True" w829 {
                tunnel: w833 -> [w841 _]
                tunnel: [w841 w842] -> w832
                tunnel: w831 -> [w840 _]
                tunnel: [w840 w843] -> w830
                tunnel: w828 -> [_ w843]
                tunnel: w827 -> [_ w842]
                frame False {
                }
                frame True {
                }
              }
            }
            frame "Step" {
              n27 = Add(x="X Reference Amplitude (nm)", y="X Reference DC Offset (nm)") -> (x+y=w866:fxp<+/-,32,16>)
              n28 = Add(x="Y Reference Amplitude (nm)", y="Y Reference DC Offset (nm)") -> (x+y=w863:fxp<+/-,32,16>)
            }
          }
          "Scan Type and Geometry" <- w817
          n29 = call "Loop Timer"("Count(uSec)"="XY Reference Loop Period (us)") -> ()  [unwired: 1 out]
          n30 = call "measure_loop_rate_FPGA.vi"() -> ("Loop Rate (Ticks)"=→"Measured XY Reference Loop Period (ticks)":u32)  [unwired: 11 in]
          n31 = xnode ("Register Write")("Data"=w819) -> ()  [unwired: 1 in, 1 out]
          n32 = xnode ("Register Write")("Data"=w822) -> ()  [unwired: 1 in, 1 out]
          n33 = xnode ("Register Write")("Data"=w821) -> ()  [unwired: 1 in, 1 out]
          "XY Reference Loop iterations" <- w824
        }
        n34 = while {
          tunnel: w104 -> [w392]
          shift-right: [w390] -> _
          shift-left: FALSE ("Data") -> [w389]
          i -> [w393]
          stop <- w391 stop-if-true
          n35 = node-c288() -> (w405:T14)  [unwired: 1 in]
          n36 = timed-loop {
            timing: w405 -> [_]
            timing-out: [_] -> w404
            tunnel: "DT Duty Cycle (periods)" -> [w416]
            tunnel: w392 -> [w415]
            tunnel: [w414] -> w400
            tunnel: "DT Reset" -> [w413]
            tunnel: "DT Phase Offset (periods)" -> [w411]
            stop <- TRUE stop-if-true
            n37 = call "Square Wave Generator2"("frequency (periods/tick)"=w415, "reset"=w413, "phase offset (periods)"=w411, "duty cycle (periods)"=w416) -> ("square wave out"=w414:bool)  [unwired: 11 in]
          }
          n38 = call "Loop Timer7"("Count(uSec)"="Trigger Generation Time Period (uSec)") -> ()  [unwired: 1 out]
          n39 = Add(x="DT Reference DC Offset (V)", y="DT Reference Amplitude (V)") -> (x+y=w397:fxp<+/-,32,16>)
          n40 = Subtract(x="DT Reference DC Offset (V)", y="DT Reference Amplitude (V)") -> (x-y=w396:fxp<+/-,32,16>)
          n41 = node-c288(w404) -> ()
          n42 = Select(t=w397, s=w400, f=w396) -> (s? t:f=w394:fxp<+/-,32,16>)
          n43 = xnode ("Register Write")("Data"=w400) -> ()  [unwired: 1 in, 1 out]
          n44 = call "measure_loop_rate_FPGA.vi"() -> ("Loop Rate (Ticks)"=→"Measured Trigger Generation Loop Period (Ticks)":u32)  [unwired: 11 in]
          n45 = xnode ("Register Read")() -> ("Data"=w390:bool)  [unwired: 1 in, 1 out]
          n46 = In Range and Coerce(upper limit="Detector Trigger Upper Limit (V)", x=w394, lower limit="Detector Trigger Lower Limit (V)") -> (coerced(x)=w395:fxp<+/-,32,16>, In Range?=→"Detector Trigger In Range?":bool)
          n47 = xnode ("Register Write")("Data"=w395) -> ()  [unwired: 1 in, 1 out]
          n48 = And(x=w390, y=w389) -> (x .and. y?=w391:bool)
          "Trigger Generation Loop iterations" <- w393
        }
        n49 = while {
          shift-right: [w379] -> _
          shift-left: FALSE ("Data") -> [w378]
          i -> [w381]
          stop <- w380 stop-if-true
          n50 = call "Loop Timer10"("Count(uSec)"="Z Reference Loop Period (us)") -> ()  [unwired: 1 out]
          n51 = Multiply(x=i16 1 ("y"), y="Z Reference Amplitude (nm)") -> (x*y=w383:fxp<+/-,56,33>)
          n52 = Add(x=w383, y="Z Reference DC Offset (nm)") -> (x+y=w382:fxp<+/-,32,16>)
          n53 = call "measure_loop_rate_FPGA.vi"() -> ("Loop Rate (Ticks)"=→"Measured Z Reference Loop Period (ticks)":u32)  [unwired: 11 in]
          n54 = xnode ("Register Read")() -> ("Data"=w379:bool)  [unwired: 1 in, 1 out]
          n55 = xnode ("Register Write")("Data"=w382) -> ()  [unwired: 1 in, 1 out]
          n56 = And(x=w379, y=w378) -> (x .and. y?=w380:bool)
          "Z Reference Loop iterations" <- w381
        }
        n57 = Equal?(x="Data Save Trigger Source", y=Data_Save_Trigger."Detector") -> (x = y?=w106:bool)
        n58 = case shown="\"Fly\", Default" w105 {
          tunnel: [w118 errorcluster {"Status?"=FALSE, "Code"=0, "Source"=""} ("error out")] -> w115
          tunnel: "Data Save Flag" -> [w117 _]
          tunnel: w106 -> [w116 _]
          frame "Fly", Default {
            n59 = case shown="\"Save Data\"" w117 {
              tunnel: [errorcluster {"Status?"=FALSE, "Code"=0, "Source"=""} ("error out") w123] -> w118
              tunnel: w116 -> [_ w122]
              frame "Skip Data", Default {
              }
              frame "Save Data" {
                n60 = while {
                  tunnel: [w126] -> w123
                  shift-right: [w136] -> _
                  shift-left: FALSE ("Data") -> [w137]
                  tunnel: w122 -> [w130]
                  shift-right: [w129] -> _
                  shift-left: FALSE ("Data") -> [w127]
                  i -> [w134]
                  stop <- w139 stop-if-true
                  n61 = Not(x=w137) -> (.not. x?=w135:bool)
                  n62 = xnode ("Register Read")() -> ("Data"=w136:bool)  [unwired: 1 in, 1 out]
                  n63 = call "Loop Timer2"("Count(uSec)"="FIFO Loop Period (us)") -> ()  [unwired: 1 out]
                  n64 = And(x=w136, y=w135) -> (x .and. y?=w132:bool)
                  n65 = Select(t=w132, s=w130, f=TRUE) -> (s? t:f=w133:bool)
                  n66 = case shown="True" w133 {
                    tunnel: [errorcluster {"Status?"=FALSE, "Code"=0, "Source"=""} ("error out") w150] -> w126
                    tunnel: [FALSE ("Status?") w149] -> w125
                    tunnel: [FALSE w148] -> w124
                    frame False {
                    }
                    frame True {
                      w167 = 5  # # of Data Strings
                      n67 = local read "Measured Controller Loop Period (Ticks)"() -> (w145:u32)
                      n68 = xnode ("Register Read")() -> ("Data"=w162:fxp<+/-,32,16>)  [unwired: 1 in, 1 out]
                      n69 = xnode ("Register Read")() -> ("Data"=w163:fxp<+/-,32,16>)  [unwired: 1 in, 1 out]
                      n70 = xnode ("Register Read")() -> ("Data"=w164:fxp<+/-,32,16>)  [unwired: 1 in, 1 out]
                      n71 = xnode ("Register Read")() -> ("Data"=w153:fxp<+/-,24,5>)  [unwired: 1 in, 1 out]
                      n72 = xnode ("Register Read")() -> ("Data"=w154:fxp<+/-,24,5>)  [unwired: 1 in, 1 out]
                      n73 = xnode ("Register Read")() -> ("Data"=w155:fxp<+/-,24,5>)  [unwired: 1 in, 1 out]
                      n74 = xnode ("Register Read")() -> ("Data"=w156:fxp<+/-,32,16>)  [unwired: 1 in, 1 out]
                      n75 = xnode ("Register Read")() -> ("Data"=w157:fxp<+/-,32,16>)  [unwired: 1 in, 1 out]
                      n76 = xnode ("Register Read")() -> ("Data"=w158:fxp<+/-,32,16>)  [unwired: 1 in, 1 out]
                      n77 = xnode ("Register Read")() -> ("Data"=w159:fxp<+/-,32,16>)  [unwired: 1 in, 1 out]
                      n78 = xnode ("Register Read")() -> ("Data"=w160:fxp<+/-,32,16>)  [unwired: 1 in, 1 out]
                      n79 = xnode ("Register Read")() -> ("Data"=w161:fxp<+/-,32,16>)  [unwired: 1 in, 1 out]
                      n80 = xnode ("Register Read")() -> ("Data"=w165:fxp<+/-,32,16>)  [unwired: 1 in, 1 out]
                      n81 = local read "Measured XY Reference Loop Period (ticks)"() -> (w144:u32)
                      n82 = case shown="\"Data Log 2\"" "Datalog Cases" {
                        tunnel: fxp<+/-,58,25> 0.0 ("fixed-point type") -> [w185 w199 w207 w219 w229 w244 w257 w268 w286 w298 w308 w320 w332 w342 w352 w365]
                        tunnel: [w193 w204 w216 w227 w240 w253 w264 w280 w290 w304 w313 w328 w339 w349 w359 w371] -> w172
                        tunnel: w162 -> [w184 _ _ _ w228 _ _ _ _ _ _ _ _ _ _ w362]
                        tunnel: w153 -> [w190 _ _ _ w233 _ _ _ _ w305 _ _ w335 _ _ _]
                        tunnel: w154 -> [_ w203 _ _ _ w248 _ _ _ _ w318 _ _ w345 _ _]
                        tunnel: w155 -> [_ _ w213 _ _ _ w261 _ _ _ _ w329 _ _ w355 _]
                        tunnel: [w192 w198 w215 w221 w239 w252 w263 w276 w289 w299 w312 w327 w338 w348 w358 w370] -> w171
                        tunnel: [w191 w205 w214 w226 w238 w251 w262 w272 w288 w300 w311 w326 w337 w347 w357 w369] -> w170
                        tunnel: w156 -> [w187 _ _ w223 w235 _ _ w283 _ w303 w317 w324 w334 _ _ w367]
                        tunnel: w157 -> [_ w200 _ w222 _ w247 _ w279 _ w302 w316 w323 _ w344 _ w366]
                        tunnel: fxp<+/-,40,17> 0.0 ("fixed-point type") -> [_ _ w209 w217 w231 w243 w255 w267 w284 w295 w307 w319 w331 w341 w351 _]
                        tunnel: w158 -> [_ _ w210 w220 _ _ w260 w275 _ w296 w315 w322 _ _ w354 _]
                        tunnel: w159 -> [_ _ _ _ w234 _ _ w282 w293 _ _ _ _ _ _ _]
                        tunnel: w160 -> [_ _ _ _ _ w246 _ w278 w292 _ _ _ _ _ _ _]
                        tunnel: w161 -> [_ _ _ _ _ _ w259 w274 w291 _ _ _ _ _ _ _]
                        tunnel: w163 -> [_ w196 _ _ _ w241 _ _ _ _ _ _ _ _ _ w361]
                        tunnel: w164 -> [_ _ w206 _ _ _ w254 _ _ _ _ _ _ _ _ _]
                        tunnel: [w189 w202 w212 w225 w237 w250 w258 w271 w287 w301 w310 w325 w336 w346 w356 w368] -> w168
                        tunnel: w167 -> [w188 w201 w211 w224 w236 w249 w265 w270 w294 w306 w314 w330 w340 w350 w360 w372]
                        tunnel: [w188 w201 w211 w224 w236 w249 w265 w270 w294 w306 w314 w330 w340 w350 w360 w372] -> w152
                        tunnel: w165 -> [_ _ _ _ _ _ _ _ _ _ _ _ _ _ _ w364]
                        tunnel: [w186 w197 w208 w218 w230 w242 w256 w269 w285 w297 w309 w321 w333 w343 w353 w363] -> w166
                        tunnel: w145 -> [w183 w195 _ _ _ _ _ _ _ _ _ _ _ _ _ _]
                        tunnel: w144 -> [w182 w194 _ _ _ _ _ _ _ _ _ _ _ _ _ _]
                        frame "Data Log 1", Default {
                          n83 = To Fixed-Point(fixed-point type=w185, number=w184) -> (fixed-point=w193:fxp<+/-,58,25>)
                          n84 = To Fixed-Point(fixed-point type=w185, number=w190) -> (fixed-point=w192:fxp<+/-,58,25>)
                          n85 = To Fixed-Point(fixed-point type=w185, number=w187) -> (fixed-point=w191:fxp<+/-,58,25>)
                          n86 = To Fixed-Point(fixed-point type=w185, number=w183) -> (fixed-point=w189:fxp<+/-,58,25>)
                          n87 = To Fixed-Point(fixed-point type=w185, number=w182) -> (fixed-point=w186:fxp<+/-,58,25>)
                        }
                        frame "Data Log 2" {
                          n88 = To Fixed-Point(fixed-point type=w199, number=w196) -> (fixed-point=w204:fxp<+/-,58,25>)
                          n89 = To Fixed-Point(fixed-point type=w199, number=w203) -> (fixed-point=w198:fxp<+/-,58,25>)
                          n90 = To Fixed-Point(fixed-point type=w199, number=w200) -> (fixed-point=w205:fxp<+/-,58,25>)
                          n91 = To Fixed-Point(fixed-point type=w199, number=w195) -> (fixed-point=w202:fxp<+/-,58,25>)
                          n92 = To Fixed-Point(fixed-point type=w199, number=w194) -> (fixed-point=w197:fxp<+/-,58,25>)
                        }
                        frame "Data Log 3" {
                          n93 = To Fixed-Point(fixed-point type=w207, number=w206) -> (fixed-point=w216:fxp<+/-,58,25>)
                          n94 = To Fixed-Point(fixed-point type=w207, number=w213) -> (fixed-point=w215:fxp<+/-,58,25>)
                          n95 = To Fixed-Point(fixed-point type=w207, number=w210) -> (fixed-point=w214:fxp<+/-,58,25>)
                          n96 = To Fixed-Point(fixed-point type=w207, number=w209) -> (fixed-point=w212:fxp<+/-,58,25>)
                          n97 = To Fixed-Point(fixed-point type=w207, number=w209) -> (fixed-point=w208:fxp<+/-,58,25>)
                        }
                        frame "Data Log 4" {
                          n98 = To Fixed-Point(fixed-point type=w219, number=w223) -> (fixed-point=w227:fxp<+/-,58,25>)
                          n99 = To Fixed-Point(fixed-point type=w219, number=w222) -> (fixed-point=w221:fxp<+/-,58,25>)
                          n100 = To Fixed-Point(fixed-point type=w219, number=w220) -> (fixed-point=w226:fxp<+/-,58,25>)
                          n101 = To Fixed-Point(fixed-point type=w219, number=w217) -> (fixed-point=w225:fxp<+/-,58,25>)
                          n102 = To Fixed-Point(fixed-point type=w219, number=w217) -> (fixed-point=w218:fxp<+/-,58,25>)
                        }
                        frame "Data Log 5" {
                          n103 = To Fixed-Point(fixed-point type=w229, number=w228) -> (fixed-point=w240:fxp<+/-,58,25>)
                          n104 = Subtract(x=w235, y=w234) -> (x-y=w232:fxp<+/-,33,17>)
                          n105 = To Fixed-Point(fixed-point type=w229, number=w233) -> (fixed-point=w239:fxp<+/-,58,25>)
                          n106 = To Fixed-Point(fixed-point type=w229, number=w232) -> (fixed-point=w238:fxp<+/-,58,25>)
                          n107 = To Fixed-Point(fixed-point type=w229, number=w231) -> (fixed-point=w237:fxp<+/-,58,25>)
                          n108 = To Fixed-Point(fixed-point type=w229, number=w231) -> (fixed-point=w230:fxp<+/-,58,25>)
                        }
                        frame "Data Log 6" {
                          n109 = To Fixed-Point(fixed-point type=w244, number=w241) -> (fixed-point=w253:fxp<+/-,58,25>)
                          n110 = To Fixed-Point(fixed-point type=w244, number=w248) -> (fixed-point=w252:fxp<+/-,58,25>)
                          n111 = Subtract(x=w247, y=w246) -> (x-y=w245:fxp<+/-,33,17>)
                          n112 = To Fixed-Point(fixed-point type=w244, number=w245) -> (fixed-point=w251:fxp<+/-,58,25>)
                          n113 = To Fixed-Point(fixed-point type=w244, number=w243) -> (fixed-point=w250:fxp<+/-,58,25>)
                          n114 = To Fixed-Point(fixed-point type=w244, number=w243) -> (fixed-point=w242:fxp<+/-,58,25>)
                        }
                        frame "Data Log 7" {
                          n115 = To Fixed-Point(fixed-point type=w257, number=w254) -> (fixed-point=w264:fxp<+/-,58,25>)
                          n116 = To Fixed-Point(fixed-point type=w257, number=w261) -> (fixed-point=w263:fxp<+/-,58,25>)
                          n117 = Subtract(x=w260, y=w259) -> (x-y=w266:fxp<+/-,33,17>)
                          n118 = To Fixed-Point(fixed-point type=w257, number=w266) -> (fixed-point=w262:fxp<+/-,58,25>)
                          n119 = To Fixed-Point(fixed-point type=w257, number=w255) -> (fixed-point=w258:fxp<+/-,58,25>)
                          n120 = To Fixed-Point(fixed-point type=w257, number=w255) -> (fixed-point=w256:fxp<+/-,58,25>)
                        }
                        frame "Data Log 8" {
                          n121 = Subtract(x=w283, y=w282) -> (x-y=w281:fxp<+/-,33,17>)
                          n122 = Subtract(x=w279, y=w278) -> (x-y=w277:fxp<+/-,33,17>)
                          n123 = To Fixed-Point(fixed-point type=w268, number=w281) -> (fixed-point=w280:fxp<+/-,58,25>)
                          n124 = Subtract(x=w275, y=w274) -> (x-y=w273:fxp<+/-,33,17>)
                          n125 = To Fixed-Point(fixed-point type=w268, number=w277) -> (fixed-point=w276:fxp<+/-,58,25>)
                          n126 = To Fixed-Point(fixed-point type=w268, number=w273) -> (fixed-point=w272:fxp<+/-,58,25>)
                          n127 = To Fixed-Point(fixed-point type=w268, number=w267) -> (fixed-point=w271:fxp<+/-,58,25>)
                          n128 = To Fixed-Point(fixed-point type=w268, number=w267) -> (fixed-point=w269:fxp<+/-,58,25>)
                        }
                        frame "Data Log 9" {
                          n129 = To Fixed-Point(fixed-point type=w286, number=w293) -> (fixed-point=w290:fxp<+/-,58,25>)
                          n130 = To Fixed-Point(fixed-point type=w286, number=w292) -> (fixed-point=w289:fxp<+/-,58,25>)
                          n131 = To Fixed-Point(fixed-point type=w286, number=w291) -> (fixed-point=w288:fxp<+/-,58,25>)
                          n132 = To Fixed-Point(fixed-point type=w286, number=w284) -> (fixed-point=w287:fxp<+/-,58,25>)
                          n133 = To Fixed-Point(fixed-point type=w286, number=w284) -> (fixed-point=w285:fxp<+/-,58,25>)
                        }
                        frame "Data Log 10" {
                          n134 = To Fixed-Point(fixed-point type=w298, number=w305) -> (fixed-point=w304:fxp<+/-,58,25>)
                          n135 = To Fixed-Point(fixed-point type=w298, number=w303) -> (fixed-point=w299:fxp<+/-,58,25>)
                          n136 = To Fixed-Point(fixed-point type=w298, number=w302) -> (fixed-point=w300:fxp<+/-,58,25>)
                          n137 = To Fixed-Point(fixed-point type=w298, number=w296) -> (fixed-point=w301:fxp<+/-,58,25>)
                          n138 = To Fixed-Point(fixed-point type=w298, number=w295) -> (fixed-point=w297:fxp<+/-,58,25>)
                        }
                        frame "Data Log 11" {
                          n139 = To Fixed-Point(fixed-point type=w308, number=w318) -> (fixed-point=w313:fxp<+/-,58,25>)
                          n140 = To Fixed-Point(fixed-point type=w308, number=w317) -> (fixed-point=w312:fxp<+/-,58,25>)
                          n141 = To Fixed-Point(fixed-point type=w308, number=w316) -> (fixed-point=w311:fxp<+/-,58,25>)
                          n142 = To Fixed-Point(fixed-point type=w308, number=w315) -> (fixed-point=w310:fxp<+/-,58,25>)
                          n143 = To Fixed-Point(fixed-point type=w308, number=w307) -> (fixed-point=w309:fxp<+/-,58,25>)
                        }
                        frame "Data Log 12" {
                          n144 = To Fixed-Point(fixed-point type=w320, number=w329) -> (fixed-point=w328:fxp<+/-,58,25>)
                          n145 = To Fixed-Point(fixed-point type=w320, number=w324) -> (fixed-point=w327:fxp<+/-,58,25>)
                          n146 = To Fixed-Point(fixed-point type=w320, number=w323) -> (fixed-point=w326:fxp<+/-,58,25>)
                          n147 = To Fixed-Point(fixed-point type=w320, number=w322) -> (fixed-point=w325:fxp<+/-,58,25>)
                          n148 = To Fixed-Point(fixed-point type=w320, number=w319) -> (fixed-point=w321:fxp<+/-,58,25>)
                        }
                        frame "Data Log 13" {
                          n149 = To Fixed-Point(fixed-point type=w332, number=w331) -> (fixed-point=w339:fxp<+/-,58,25>)
                          n150 = To Fixed-Point(fixed-point type=w332, number=w335) -> (fixed-point=w338:fxp<+/-,58,25>)
                          n151 = To Fixed-Point(fixed-point type=w332, number=w334) -> (fixed-point=w337:fxp<+/-,58,25>)
                          n152 = To Fixed-Point(fixed-point type=w332, number=w331) -> (fixed-point=w336:fxp<+/-,58,25>)
                          n153 = To Fixed-Point(fixed-point type=w332, number=w331) -> (fixed-point=w333:fxp<+/-,58,25>)
                        }
                        frame "Data Log 14" {
                          n154 = To Fixed-Point(fixed-point type=w342, number=w341) -> (fixed-point=w349:fxp<+/-,58,25>)
                          n155 = To Fixed-Point(fixed-point type=w342, number=w345) -> (fixed-point=w348:fxp<+/-,58,25>)
                          n156 = To Fixed-Point(fixed-point type=w342, number=w344) -> (fixed-point=w347:fxp<+/-,58,25>)
                          n157 = To Fixed-Point(fixed-point type=w342, number=w341) -> (fixed-point=w346:fxp<+/-,58,25>)
                          n158 = To Fixed-Point(fixed-point type=w342, number=w341) -> (fixed-point=w343:fxp<+/-,58,25>)
                        }
                        frame "Data Log 15" {
                          n159 = To Fixed-Point(fixed-point type=w352, number=w351) -> (fixed-point=w359:fxp<+/-,58,25>)
                          n160 = To Fixed-Point(fixed-point type=w352, number=w355) -> (fixed-point=w358:fxp<+/-,58,25>)
                          n161 = To Fixed-Point(fixed-point type=w352, number=w354) -> (fixed-point=w357:fxp<+/-,58,25>)
                          n162 = To Fixed-Point(fixed-point type=w352, number=w351) -> (fixed-point=w356:fxp<+/-,58,25>)
                          n163 = To Fixed-Point(fixed-point type=w352, number=w351) -> (fixed-point=w353:fxp<+/-,58,25>)
                        }
                        frame "Data Log 16" {
                          n164 = To Fixed-Point(fixed-point type=w365, number=w362) -> (fixed-point=w371:fxp<+/-,58,25>)
                          n165 = To Fixed-Point(fixed-point type=w365, number=w361) -> (fixed-point=w370:fxp<+/-,58,25>)
                          n166 = To Fixed-Point(fixed-point type=w365, number=w367) -> (fixed-point=w369:fxp<+/-,58,25>)
                          n167 = To Fixed-Point(fixed-point type=w365, number=w366) -> (fixed-point=w368:fxp<+/-,58,25>)
                          n168 = To Fixed-Point(fixed-point type=w365, number=w364) -> (fixed-point=w363:fxp<+/-,58,25>)
                        }
                      }
                      "Number of Data Strings" <- w152
                      n169 = Build Array(w172, w171, w170, w168, w166) -> (w151:fxp<+/-,58,25>[])
                      n170 = for {
                        N: w152 -> [_]
                        tunnel: w151 -> [w181] mode=indexing
                        shift-right: [w179] -> w150
                        shift-left: errorcluster {"Status?"=FALSE, "Code"=0, "Source"=""} ("error out") -> [w178]
                        shift-right: [w175] -> w148
                        shift-left: FALSE -> [w176]
                        n171 = xnode ("FIFO")("Element"=w181, "Timeout"="Timeout FPGA FIFO1", "error in (no error)"=w178) -> ("Timed Out?"=w177:bool, "error out"=w179:errorcluster)  [unwired: 1 in, 1 out]
                        "FIFO Timed Out?" <- w177
                        n172 = Or(x=w177, y=w176) -> (x .or. y?=w175:bool)
                      }
                      "FIFO Timed Out" <- w148
                      n173 = Unbundle By Name(w150) -> ("Status?"=w149:bool)
                    }
                  }
                  n174 = xnode ("Register Read")() -> ("Data"=w129:bool)  [unwired: 1 in, 1 out]
                  n175 = call "measure_loop_rate_FPGA.vi"() -> ("Loop Rate (Ticks)"=→"Measured Datalog Period (Ticks)":u32)  [unwired: 11 in]
                  n176 = And(x=w127, y=w129) -> (x .and. y?=w128:bool)
                  n177 = Compound Arithmetic op=OR(w125, w124, w128) -> (w139:bool)
                  n178 = case shown="True" w139 {
                    selector: w139 -> [_ w373]
                    frame False {
                    }
                    frame True {
                      n179 = xnode ("Register Write")("Data"=w373) -> ()  [unwired: 1 in, 1 out]
                      n180 = local write "Stop Scan"(w373) -> ()
                    }
                  }
                  "FIFO loop iterations" <- w134
                }
              }
            }
          }
          frame "Step" {
          }
        }
        n181 = while {
          shift-right: [w475] -> _
          shift-left: _ -> [w466]
          shift-right: [w474] -> _
          shift-left: _ -> [w465]
          shift-right: [w473] -> _
          shift-left: _ -> [w464]
          shift-right: [w472] -> _
          shift-left: _ -> [w463]
          shift-right: [w471] -> _
          shift-left: _ -> [w462]
          shift-right: [w470] -> _
          shift-left: _ -> [w461]
          shift-right: [w469] -> _
          shift-left: _ -> [w460]
          shift-right: [w468] -> _
          shift-left: _ -> [w459]
          shift-right: [w467] -> _
          shift-left: _ -> [w458]
          shift-right: [w435] -> _
          shift-left: FALSE ("Data") -> [w434]
          i -> [w443]
          stop <- w436 stop-if-true
          n182 = xnode ("Register Read")() -> ("Data"=w448:fxp<+/-,32,16>)  [unwired: 1 in, 1 out]
          n183 = xnode ("Register Read")() -> ("Data"=w446:fxp<+/-,32,16>)  [unwired: 1 in, 1 out]
          n184 = xnode ("Register Read")() -> ("Data"=w444:fxp<+/-,32,16>)  [unwired: 1 in, 1 out]
          n185 = xnode ("Register Read")() -> ("Data"=w449:fxp<+/-,32,16>)  [unwired: 1 in, 1 out]
          n186 = xnode ("Register Read")() -> ("Data"=w447:fxp<+/-,32,16>)  [unwired: 1 in, 1 out]
          n187 = xnode ("Register Read")() -> ("Data"=w445:fxp<+/-,32,16>)  [unwired: 1 in, 1 out]
          n188 = xnode ("Register Read")() -> ("Data"=w452:fxp<+/-,32,16>)  [unwired: 1 in, 1 out]
          n189 = xnode ("Register Read")() -> ("Data"=w451:fxp<+/-,32,16>)  [unwired: 1 in, 1 out]
          n190 = xnode ("Register Read")() -> ("Data"=w450:fxp<+/-,32,16>)  [unwired: 1 in, 1 out]
          n191 = call "Loop Timer3"("Count(uSec)"="Controller Loop Period (uSec)") -> ()  [unwired: 1 out]
          n192 = case shown="\"Optics Stage Only\", Default" "Optics and or Sample Stage" {
            tunnel: w448 -> [_ w494]
            tunnel: w449 -> [w485 w493]
            tunnel: [w485 w492] -> w457
            tunnel: w446 -> [_ w491]
            tunnel: w447 -> [w484 w490]
            tunnel: [w484 w489] -> w456
            tunnel: w444 -> [_ w488]
            tunnel: w445 -> [w483 w487]
            tunnel: [w483 w486] -> w455
            frame "Optics Stage Only", Default {
            }
            frame "Optics and Sample Stage" {
              n193 = Subtract(x=w493, y=w494) -> (x-y=w492:fxp<+/-,33,17>)
              n194 = Subtract(x=w490, y=w491) -> (x-y=w489:fxp<+/-,33,17>)
              n195 = Subtract(x=w487, y=w488) -> (x-y=w486:fxp<+/-,33,17>)
            }
          }
          n196 = case shown="\"Closed Loop\"" "System Loop Type" {
            tunnel: w457 -> [_ w544]
            tunnel: w452 -> [w500 w516]
            tunnel: [w496 w513] -> w438
            tunnel: [w497 w511] -> w439
            tunnel: [_ w543] -> w475
            tunnel: [_ w542] -> w474
            tunnel: [_ w541] -> w473
            tunnel: [_ w540] -> w472
            tunnel: [_ w539] -> w471
            tunnel: [_ w538] -> w470
            tunnel: [_ w537] -> w469
            tunnel: [_ w536] -> w468
            tunnel: [_ w535] -> w467
            tunnel: w465 -> [_ w534]
            tunnel: w464 -> [_ w533]
            tunnel: w463 -> [_ w532]
            tunnel: w462 -> [_ w531]
            tunnel: w461 -> [_ w530]
            tunnel: w460 -> [_ w529]
            tunnel: w459 -> [_ w528]
            tunnel: w458 -> [_ w527]
            tunnel: w456 -> [_ w526]
            tunnel: w451 -> [w499 w515]
            tunnel: w450 -> [w498 w514]
            tunnel: w455 -> [_ w523]
            tunnel: [w495 w512] -> w437
            tunnel: w466 -> [_ w525]
            frame "Open Loop", Default {
              n197 = Multiply(x="X-Stage nm to V Scaling", y="X-Stage Scaling Direction") -> (x*y=w508:fxp<+/-,35,15>)
              n198 = Multiply(x="Y-Stage nm to V Scaling", y="Y-Stage Scaling Direction") -> (x*y=w504:fxp<+/-,35,15>)
              n199 = Multiply(x="Z-Stage nm to V Scaling", y="Z-Stage Scaling Direction") -> (x*y=w503:fxp<+/-,35,15>)
              n200 = Multiply(x=w500, y=w508) -> (x*y=w497:fxp<+/-,32,16>)
              n201 = Multiply(x=w499, y=w504) -> (x*y=w496:fxp<+/-,32,16>)
              n202 = Multiply(x=w498, y=w503) -> (x*y=w495:fxp<+/-,32,16>)
            }
            frame "Closed Loop" {
              w520 = fxp<+/-,58,25> 0.0 ("fixed-point type")
              n203 = Subtract(x=w516, y=w544) -> (x-y=w548:fxp<+/-,34,18>)
              n204 = Subtract(x=w515, y=w526) -> (x-y=w547:fxp<+/-,34,18>)
              n205 = Subtract(x=w514, y=w523) -> (x-y=w524:fxp<+/-,34,18>)
              n206 = To Fixed-Point(fixed-point type=w520, number=w548) -> (fixed-point=w546:fxp<+/-,58,25>)
              n207 = To Fixed-Point(fixed-point type=w520, number=w547) -> (fixed-point=w545:fxp<+/-,58,25>)
              n208 = To Fixed-Point(fixed-point type=w520, number=w524) -> (fixed-point=w522:fxp<+/-,58,25>)
              n209 = for {
                N: 3 -> [_]
                shift-right: [w626] -> w519
                shift-left: _ -> [w624]
                shift-right: [w623] -> w518
                shift-left: _ -> [w621]
                tunnel: [w614] -> w543
                shift-right: [w613] -> _
                shift-left: _ -> [w609]
                tunnel: [w612] -> w542
                shift-right: [w611] -> _
                shift-left: _ -> [w607]
                tunnel: w525 -> [w604]
                tunnel: w534 -> [w603]
                tunnel: [w602] -> w540
                shift-right: [w601] -> _
                shift-left: _ -> [w594]
                tunnel: [w600] -> w539
                shift-right: [w599] -> _
                shift-left: _ -> [w593]
                tunnel: [w598] -> w537
                tunnel: [w597] -> w536
                shift-right: [w596] -> _
                shift-left: _ -> [w592]
                shift-right: [w595] -> _
                shift-left: _ -> [w581]
                tunnel: w532 -> [w591]
                tunnel: w531 -> [w590]
                tunnel: w529 -> [w589]
                tunnel: w528 -> [w588]
                tunnel: w546 -> [w580]
                tunnel: w545 -> [w577]
                shift-right: [w576] -> w517
                shift-left: _ -> [w573]
                tunnel: [w568] -> w541
                tunnel: [w567] -> w538
                tunnel: [w566] -> w535
                shift-right: [w565] -> _
                shift-left: _ -> [w561]
                shift-right: [w564] -> _
                shift-left: _ -> [w559]
                shift-right: [w563] -> _
                shift-left: _ -> [w557]
                tunnel: w533 -> [w556]
                tunnel: w527 -> [w555]
                tunnel: w530 -> [w554]
                tunnel: w522 -> [w550]
                i -> [w631]
                # "ez"
                # "ey"
                # "ex"
                n210 = Add(x=1, y=w631) -> (x+y=w549:i32)
                n211 = flat-sequence {
                  tunnel: [w674] -> w641
                  tunnel: [w673] -> w640
                  tunnel: [w672] -> w639
                  tunnel: [w671] -> w638
                  tunnel: [w670] -> w637
                  tunnel: [w669] -> w636
                  tunnel: [w668] -> w635
                  tunnel: [w667] -> w634
                  tunnel: w549 -> [w675]
                  tunnel: [w653] -> w633
                  tunnel: [w666] -> w625
                  tunnel: w624 -> [w666]
                  tunnel: [w665] -> w622
                  tunnel: w621 -> [w665]
                  tunnel: [w664] -> w610
                  tunnel: w609 -> [w664]
                  tunnel: [w644] -> w608
                  tunnel: w607 -> [w644]
                  tunnel: w604 -> [w655]
                  tunnel: w603 -> [w656]
                  tunnel: w594 -> [w663]
                  tunnel: w593 -> [w662]
                  tunnel: w592 -> [w661]
                  tunnel: w591 -> [w657]
                  tunnel: w590 -> [w658]
                  tunnel: w589 -> [w659]
                  tunnel: w588 -> [w660]
                  tunnel: w581 -> [w654]
                  tunnel: [w663] -> w587
                  tunnel: [w662] -> w586
                  tunnel: [w661] -> w585
                  tunnel: w580 -> [w643]
                  tunnel: [w654] -> w579
                  tunnel: w577 -> [w642]
                  tunnel: [w652] -> w574
                  tunnel: w573 -> [w652]
                  tunnel: [w651] -> w562
                  tunnel: w561 -> [w651]
                  tunnel: [w650] -> w560
                  tunnel: w559 -> [w650]
                  tunnel: [w649] -> w558
                  tunnel: w557 -> [w649]
                  tunnel: w556 -> [w646]
                  tunnel: w555 -> [w648]
                  tunnel: w554 -> [w647]
                  tunnel: w550 -> [w645]
                  tunnel: w641 -> [w727]
                  tunnel: w640 -> [w726]
                  tunnel: w639 -> [w725]
                  tunnel: w638 -> [w705]
                  tunnel: w637 -> [w706]
                  tunnel: w636 -> [w707]
                  tunnel: w635 -> [w708]
                  tunnel: w634 -> [w709]
                  tunnel: w633 -> [w714]
                  tunnel: [w712] -> w630
                  tunnel: [w712] -> w629
                  tunnel: [w703] -> w628
                  tunnel: [w704] -> w627
                  tunnel: w625 -> [w704]
                  tunnel: w622 -> [w703]
                  tunnel: [w713] -> w620
                  tunnel: [w713] -> w619
                  tunnel: [w711] -> w618
                  tunnel: [w711] -> w617
                  tunnel: [w710] -> w616
                  tunnel: [w710] -> w615
                  tunnel: w610 -> [w724]
                  tunnel: w608 -> [w723]
                  tunnel: [w724] -> w606
                  tunnel: [w723] -> w605
                  tunnel: w587 -> [w722]
                  tunnel: w586 -> [w721]
                  tunnel: w585 -> [w720]
                  tunnel: [w722] -> w584
                  tunnel: [w721] -> w583
                  tunnel: [w720] -> w582
                  tunnel: w579 -> [w719]
                  tunnel: [w719] -> w578
                  tunnel: [w712] -> w575
                  tunnel: w574 -> [w718]
                  tunnel: [w718] -> w572
                  tunnel: [w713] -> w571
                  tunnel: [w711] -> w570
                  tunnel: [w710] -> w569
                  tunnel: w562 -> [w717]
                  tunnel: w560 -> [w716]
                  tunnel: w558 -> [w715]
                  tunnel: [w717] -> w553
                  tunnel: [w716] -> w552
                  tunnel: [w715] -> w551
                  tunnel: w630 -> [w755]
                  tunnel: w629 -> [w810]
                  tunnel: w549 -> [w754]
                  tunnel: w628 -> [w809]
                  tunnel: w627 -> [w756]
                  tunnel: [w759] -> w626
                  tunnel: [w758] -> w623
                  tunnel: w620 -> [w796]
                  tunnel: w619 -> [w795]
                  tunnel: w618 -> [w794]
                  tunnel: w617 -> [w793]
                  tunnel: w616 -> [w792]
                  tunnel: w615 -> [w791]
                  tunnel: [w790] -> w614
                  tunnel: [w790] -> w613
                  tunnel: [w789] -> w612
                  tunnel: [w789] -> w611
                  tunnel: w606 -> [w788]
                  tunnel: w605 -> [w787]
                  tunnel: [w786] -> w602
                  tunnel: [w786] -> w601
                  tunnel: [w785] -> w600
                  tunnel: [w785] -> w599
                  tunnel: [w784] -> w598
                  tunnel: [w783] -> w597
                  tunnel: [w784] -> w596
                  tunnel: [w783] -> w595
                  tunnel: w584 -> [w782]
                  tunnel: w583 -> [w781]
                  tunnel: w582 -> [w780]
                  tunnel: w578 -> [w779]
                  tunnel: [w757] -> w576
                  tunnel: w575 -> [w776]
                  tunnel: w572 -> [w775]
                  tunnel: w571 -> [w768]
                  tunnel: w570 -> [w767]
                  tunnel: w569 -> [w766]
                  tunnel: [w765] -> w568
                  tunnel: [w764] -> w567
                  tunnel: [w763] -> w566
                  tunnel: [w765] -> w565
                  tunnel: [w764] -> w564
                  tunnel: [w763] -> w563
                  tunnel: w553 -> [w762]
                  tunnel: w552 -> [w761]
                  tunnel: w551 -> [w760]
                  frame #0 {
                    n212 = case shown="1, Default" w675 {
                      tunnel: ["sos gain SF Controller xx1" "sos gain SF Controller yy1" "sos gain SF Controller zz1"] -> w671
                      tunnel: ["-a01(2) xx1" "-a01(2) yy1" "-a01(2) zz1"] -> w670
                      tunnel: ["-a02(2) xx1" "-a02(2) yy1" "-a02(2) zz1"] -> w669
                      tunnel: ["b01(2) xx1" "b01(2) yy1" "b01(2) zz1"] -> w668
                      tunnel: ["b02(2) xx1" "b02(2) yy1" "b02(2) zz1"] -> w667
                      tunnel: [w676 w687 w701] -> w672
                      tunnel: [w682 w686 w700] -> w673
                      tunnel: [w683 w685 w699] -> w674
                      tunnel: w655 -> [w683 _ _]
                      tunnel: w656 -> [_ w685 _]
                      tunnel: w657 -> [w682 _ _]
                      tunnel: w658 -> [_ w686 _]
                      tunnel: w659 -> [w676 _ _]
                      tunnel: w660 -> [_ w687 _]
                      tunnel: [w684 w693 w702] -> w653
                      tunnel: w643 -> [w684 _ _]
                      tunnel: w642 -> [_ w693 _]
                      tunnel: w648 -> [_ _ w701]
                      tunnel: w647 -> [_ _ w700]
                      tunnel: w646 -> [_ _ w699]
                      tunnel: w645 -> [_ _ w702]
                      frame 1, Default {
                      }
                      frame 2 {
                      }
                      frame 3 {
                      }
                    }
                  }
                  frame #1 {
                    # "n_i"
                    # "m_i"
                    # "l_i"
                    # "u_i"
                    n213 = Multiply(x=w714, y=w705) -> (x*y=w728:fxp<+/-,64,34>)
                    n214 = To Fixed-Point(number=w728) -> (fixed-point=w729:fxp<+/-,58,25>)  [unwired: 1 in]
                    n215 = for {
                      tunnel: w706 -> [w746] mode=indexing
                      tunnel: w709 -> [w743] mode=indexing
                      shift-right: [w748] -> w712
                      shift-left: w729 -> [w747]
                      tunnel: w707 -> [w745] mode=indexing
                      tunnel: w708 -> [w744] mode=indexing
                      tunnel: [w735] -> w713 mode=indexing
                      tunnel: w727 -> [w741] mode=indexing
                      tunnel: [w738] -> w711 mode=indexing
                      tunnel: w726 -> [w731] mode=indexing
                      tunnel: [w731] -> w710 mode=indexing
                      tunnel: w725 -> [w739] mode=indexing
                      # "b_1"
                      # "b_2"
                      # "n_i-1"
                      # "-a_2"
                      # "-a_1"
                      # "m_i-1"
                      # "l_i-1"
                      # "e_i"
                      n216 = To Fixed-Point(number=w741) -> (fixed-point=w753:fxp<+/-,58,25>)  [unwired: 1 in]
                      n217 = Add(x=w747, y=w753) -> (x+y=w740:fxp<+/-,59,26>)
                      n218 = To Fixed-Point(number=w740) -> (fixed-point=w738:fxp<+/-,58,25>)  [unwired: 1 in]
                      n219 = Multiply(x=w738, y=w746) -> (x*y=w730:fxp<+/-,64,34>)
                      n220 = Multiply(x=w739, y=w743) -> (x*y=w752:fxp<+/-,64,34>)
                      n221 = Multiply(x=w731, y=w745) -> (x*y=w749:fxp<+/-,64,34>)
                      n222 = To Fixed-Point(number=w730) -> (fixed-point=w734:fxp<+/-,58,25>)  [unwired: 1 in]
                      n223 = To Fixed-Point(number=w749) -> (fixed-point=w733:fxp<+/-,58,25>)  [unwired: 1 in]
                      n224 = To Fixed-Point(number=w752) -> (fixed-point=w732:fxp<+/-,58,25>)  [unwired: 1 in]
                      n225 = Add(x=w734, y=w733) -> (x+y=w742:fxp<+/-,59,26>)
                      n226 = To Fixed-Point(number=w742) -> (fixed-point=w735:fxp<+/-,58,25>)  [unwired: 1 in]
                      n227 = Multiply(x=w731, y=w744) -> (x*y=w750:fxp<+/-,64,34>)
                      n228 = To Fixed-Point(number=w750) -> (fixed-point=w736:fxp<+/-,58,25>)  [unwired: 1 in]
                      n229 = Add(x=w736, y=w732) -> (x+y=w751:fxp<+/-,59,26>)
                      n230 = To Fixed-Point(number=w751) -> (fixed-point=w737:fxp<+/-,58,25>)  [unwired: 1 in]
                      n231 = Add(x=w738, y=w737) -> (x+y=w748:fxp<+/-,58,25>)
                    }
                  }
                  frame #2 {
                    n232 = Equal?(x=3, y=w754) -> (x = y?=w777:bool)
                    n233 = Equal?(x=2, y=w754) -> (x = y?=w811:bool)
                    n234 = Equal?(x=1, y=w754) -> (x = y?=w813:bool)
                    n235 = Equal?(x=2, y=w754) -> (x = y?=w801:bool)
                    n236 = Equal?(x=2, y=w754) -> (x = y?=w805:bool)
                    n237 = Equal?(x=3, y=w754) -> (x = y?=w773:bool)
                    n238 = Equal?(x=2, y=w754) -> (x = y?=w797:bool)
                    n239 = Equal?(x=1, y=w754) -> (x = y?=w807:bool)
                    n240 = Equal?(x=1, y=w754) -> (x = y?=w803:bool)
                    n241 = Equal?(x=3, y=w754) -> (x = y?=w771:bool)
                    n242 = Equal?(x=1, y=w754) -> (x = y?=w799:bool)
                    n243 = Equal?(x=3, y=w754) -> (x = y?=w769:bool)
                    n244 = Select(t=w776, s=w777, f=w775) -> (s? t:f=w757:fxp<+/-,58,25>)
                    "Kzz Output, Kzz*ez (V)" <- w757
                    n245 = Select(t=w810, s=w811, f=w809) -> (s? t:f=w758:fxp<+/-,58,25>)
                    "Kyy Output, Kyy*ey (V)" <- w758
                    n246 = Select(t=w755, s=w813, f=w756) -> (s? t:f=w759:fxp<+/-,58,25>)
                    "Kxx Output, Kxx*ex (V)" <- w759
                    n247 = Select(t=w793, s=w801, f=w781) -> (s? t:f=w785:fxp<+/-,58,25>[])
                    n248 = Select(t=w795, s=w805, f=w787) -> (s? t:f=w789:fxp<+/-,58,25>[])
                    n249 = Select(t=w768, s=w773, f=w762) -> (s? t:f=w765:fxp<+/-,58,25>[])
                    n250 = Select(t=w791, s=w797, f=w779) -> (s? t:f=w783:fxp<+/-,58,25>[])
                    n251 = Select(t=w796, s=w807, f=w788) -> (s? t:f=w790:fxp<+/-,58,25>[])
                    n252 = Select(t=w794, s=w803, f=w782) -> (s? t:f=w786:fxp<+/-,58,25>[])
                    n253 = Select(t=w767, s=w771, f=w761) -> (s? t:f=w764:fxp<+/-,58,25>[])
                    n254 = Select(t=w792, s=w799, f=w780) -> (s? t:f=w784:fxp<+/-,58,25>[])
                    n255 = Select(t=w766, s=w769, f=w760) -> (s? t:f=w763:fxp<+/-,58,25>[])
                  }
                }
              }
              n256 = Multiply(x=w517, y="Scaling mV to V") -> (x*y=w512:fxp<+/-,32,16>)
              n257 = Multiply(x=w519, y="Scaling mV to V") -> (x*y=w511:fxp<+/-,32,16>)
              n258 = Multiply(x=w518, y="Scaling mV to V") -> (x*y=w513:fxp<+/-,32,16>)
            }
          }
          n259 = xnode ("Register Read")() -> ("Data"=w435:bool)  [unwired: 1 in, 1 out]
          n260 = call "measure_loop_rate_FPGA.vi"() -> ("Loop Rate (Ticks)"=→"Measured Controller Loop Period (Ticks)":u32)  [unwired: 11 in]
          n261 = In Range and Coerce(upper limit="Controller Output Upper Limit", x=w439, lower limit="Controller Output Lower Limit") -> (coerced(x)=w442:fxp<+/-,32,16>, In Range?=→"X-Stage Input In Range?":bool)
          n262 = In Range and Coerce(upper limit="Controller Output Upper Limit", x=w437, lower limit="Controller Output Lower Limit") -> (coerced(x)=w440:fxp<+/-,32,16>, In Range?=→"Z-Stage Input In Range?":bool)
          n263 = In Range and Coerce(upper limit="Controller Output Upper Limit", x=w438, lower limit="Controller Output Lower Limit") -> (coerced(x)=w441:fxp<+/-,32,16>, In Range?=→"Y-Stage Input In Range?":bool)
          n264 = xnode ("Register Write")("Data"=w441) -> ()  [unwired: 1 in, 1 out]
          n265 = xnode ("Register Write")("Data"=w442) -> ()  [unwired: 1 in, 1 out]
          n266 = xnode ("Register Write")("Data"=w440) -> ()  [unwired: 1 in, 1 out]
          n267 = And(x=w435, y=w434) -> (x .and. y?=w436:bool)
          "Controller loop iterations" <- w443
        }
        n268 = while {
          tunnel: [w430] -> w111
          shift-right: [w422] -> _
          shift-left: FALSE ("Data") -> [w421]
          i -> [w424]
          stop <- w432 stop-if-true
          n269 = xnode ("Register Read")() -> ("Data"=w425:fxp<+/-,32,16>)  [unwired: 1 in, 1 out]
          n270 = xnode ("Register Read")() -> ("Data"=w428:fxp<+/-,24,5>)  [unwired: 1 in, 1 out]
          n271 = xnode ("Register Read")() -> ("Data"=w427:fxp<+/-,24,5>)  [unwired: 1 in, 1 out]
          n272 = xnode ("Register Read")() -> ("Data"=w426:fxp<+/-,24,5>)  [unwired: 1 in, 1 out]
          n273 = xnode "FPGA I/O Node"("Mod8/AO0"=w428, "Mod8/AO1"=w427, "Mod8/AO2"=w426, "Mod8/AO3"=w425) -> ("error out"=w430:errorcluster)  [unwired: 5 in, 4 out]
          n274 = call "Loop Timer4"("Count(uSec)"="Module Output Loop Period (uSec)") -> ()  [unwired: 1 out]
          n275 = xnode ("Register Read")() -> ("Data"=w422:bool)  [unwired: 1 in, 1 out]
          n276 = call "measure_loop_rate_FPGA.vi"() -> ("Loop Rate (Ticks)"=→"Measured Module Output Loop Period (Ticks)":u32)  [unwired: 11 in]
          n277 = Unbundle By Name(w430) -> ("status"=w431:bool)
          n278 = And(x=w422, y=w421) -> (x .and. y?=w423:bool)
          n279 = Or(x=w431, y=w423) -> (x .or. y?=w432:bool)
          "Module output loop iterations" <- w424
        }
        n280 = Merge Errors(w111, w115) -> (w112:errorcluster)
        "Run Loop error" <- w112
        n281 = case shown="Error" w112 {
          tunnel: [FPGA_states."End Run" FPGA_states."Wait"] -> w113
          frame No Error {
          }
          frame Error {
            n282 = local write "Stop Scan"(TRUE) -> ()
          }
        }
      }
      frame "End Run" {
        n283 = flat-sequence {
          tunnel: w871 -> [w874]
          tunnel: [w874] -> w870
          frame #0 {
            n284 = xnode ("Register Write")("Data"=FALSE) -> ()  [unwired: 1 in, 1 out]
          }
        }
        "End Run Error" <- w871
      }
      frame "Shutdown" {
        n285 = xnode "FPGA I/O Node"("error in"=w878, "System Reset"=TRUE) -> ("error out"=w877:errorcluster)  [unwired: 1 in, 1 out]
        "Shutdown error" <- w877
      }
    }
    "FPGA state" <- w20
    "Outer Loop iterations" <- w11
  }
  n286 = while {
    tunnel: w1 -> [w894]
    shift-right: [w892] -> _
    shift-left: _ -> [w891]
    shift-right: [w889] -> _
    shift-left: u8 0 ("USER FPGA LED") -> [w887]
    stop <- FALSE stop-if-true
    # "Heartbeat Loop - monitors errors and relays status to RT and LED on cRIO"
    n287 = local read "Interferometer Loop Error"() -> (w881:errorcluster)
    n288 = local read "Shutdown error"() -> (w896:errorcluster)
    n289 = local read "Run Loop error"() -> (w899:errorcluster)
    n290 = local read "Start Run Error"() -> (w898:errorcluster)
    n291 = local read "End Run Error"() -> (w895:errorcluster)
    n292 = local read "Wait error"() -> (w897:errorcluster)
    n293 = Merge Errors(w891, w899, w898, w897, w896, w895, w881, w894) -> (w893:errorcluster)
    "FPGA error monitor" <- w893
    n294 = Unbundle By Name(w893) -> ("status"=w882:bool)
    n295 = Not Equal?(x=w887, y=u8 0) -> (x != y?=w885:bool)
    n296 = case shown="False" w882 {
      tunnel: [u16 500 ("Count(mSec)") u16 100 ("Count(mSec)")] -> w890
      tunnel: [u8 1 ("USER FPGA LED") u8 2 ("USER FPGA LED")] -> w883
      frame False {
        # "Set LED green \nand rep rate to 1 Hz"
      }
      frame True {
        # "Set LED yellow \nand rep rate to 5 Hz"
      }
    }
    n297 = Select(t=u8 0, s=w885, f=w883) -> (s? t:f=w889:u8)
    n298 = xnode "FPGA I/O Node"("USER FPGA LED"=w889) -> ("error out"=w892:errorcluster)  [unwired: 2 in, 1 out]
    n299 = call "Loop Timer12"("Count(mSec)"=w890) -> ()  [unwired: 1 out]
  }
  n300 = while {
    i -> [w904]
    stop <- FALSE stop-if-true
    n301 = xnode ("Register Read")() -> ("Data"=w908:i32)  [unwired: 1 in, 1 out]
    n302 = xnode ("Register Read")() -> ("Data"=w909:i32)  [unwired: 1 in, 1 out]
    n303 = xnode ("Register Read")() -> ("Data"=w910:i32)  [unwired: 1 in, 1 out]
    n304 = xnode ("Register Read")() -> ("Data"=w905:i32)  [unwired: 1 in, 1 out]
    n305 = xnode ("Register Read")() -> ("Data"=w906:i32)  [unwired: 1 in, 1 out]
    n306 = xnode ("Register Read")() -> ("Data"=w907:i32)  [unwired: 1 in, 1 out]
    n307 = call "Loop Timer5"("Count(uSec)"="Plant Output Loop Period (uSec)") -> ()  [unwired: 1 out]
    n308 = call "measure_loop_rate_FPGA.vi"() -> ("Loop Rate (Ticks)"=→"Measured Plant Output Loop Period (Ticks)":u32)  [unwired: 11 in]
    n309 = Multiply(x=w905, y="Optics X Stage Resolution (nm)") -> (x*y=w923:fxp<+/-,32,16>)
    "Optics X Stage Displacement raw (nm)" <- w923
    n310 = Multiply(x=w908, y="Sample X Stage Resolution (nm)") -> (x*y=w917:fxp<+/-,32,16>)
    "Sample X Stage Displacement raw (nm)" <- w917
    n311 = Multiply(x=w906, y="Optics Y Stage Resolution (nm)") -> (x*y=w920:fxp<+/-,32,16>)
    "Optics Y Stage Displacement raw (nm)" <- w920
    n312 = Multiply(x=w909, y="Sample Y Stage Resolution (nm)") -> (x*y=w916:fxp<+/-,32,16>)
    "Sample Y Stage Displacement raw (nm)" <- w916
    n313 = Multiply(x=w907, y="Optics Z Stage Resolution (nm)") -> (x*y=w918:fxp<+/-,32,16>)
    "Optics Z Stage Displacement raw (nm)" <- w918
    n314 = Multiply(x=w910, y="Sample Z Stage Resolution (nm)") -> (x*y=w915:fxp<+/-,32,16>)
    "Sample Z Stage Displacement raw (nm)" <- w915
    n315 = xnode ("Register Write")("Data"=w923) -> ()  [unwired: 1 in, 1 out]
    n316 = xnode ("Register Write")("Data"=w920) -> ()  [unwired: 1 in, 1 out]
    n317 = xnode ("Register Write")("Data"=w918) -> ()  [unwired: 1 in, 1 out]
    n318 = xnode ("Register Write")("Data"=w917) -> ()  [unwired: 1 in, 1 out]
    n319 = xnode ("Register Write")("Data"=w916) -> ()  [unwired: 1 in, 1 out]
    n320 = xnode ("Register Write")("Data"=w915) -> ()  [unwired: 1 in, 1 out]
    "Plant output loop iterations" <- w904
  }
  n321 = node-c288(refnum<k21> "40 MHz Onboard Clock" ("Source Name"), w1) -> (w6:T14)
  n322 = timed-loop {
    timing: w6 -> [_]
    timing-out: [_] -> w5
    shift-right: [w964] -> _
    shift-left: _ -> [w966]
    shift-right: [w963] -> _
    shift-left: _ -> [w965]
    shift-right: [w930] -> _
    shift-left: w4 -> [w977]
    shift-right: [w979] -> _
    shift-left: u32 0 ("Tick Count(Ticks)") -> [w978]
    shift-right: [w955] -> _
    shift-left: _ -> [w954]
    shift-right: [w956] -> _
    shift-left: _ -> [w953]
    shift-right: [w932] -> _
    shift-left: w4 -> [w974]
    shift-right: [w943] -> _
    shift-left: _ -> [w944]
    shift-right: [w942] -> _
    shift-left: _ -> [w945]
    shift-right: [w928] -> _
    shift-left: w4 -> [w970]
    shift-right: [w961] -> _
    shift-left: _ -> [w959]
    shift-right: [w960] -> _
    shift-left: _ -> [w958]
    shift-right: [w931] -> _
    shift-left: w4 -> [w976]
    shift-right: [w948] -> _
    shift-left: _ -> [w949]
    shift-right: [w947] -> _
    shift-left: _ -> [w950]
    shift-right: [w929] -> _
    shift-left: w4 -> [w972]
    shift-right: [w938] -> _
    shift-left: _ -> [w940]
    shift-right: [w939] -> _
    shift-left: _ -> [w941]
    shift-right: [w927] -> _
    shift-left: w4 -> [w968]
    shift-right: [w935] -> _
    shift-left: _ -> [w934]
    i -> [w926]
    stop <- w933 stop-if-true
    # "Tracks interferometer data"
    n323 = xnode "FPGA I/O Node"("error in"=w934) -> ("error out"=w957:errorcluster, "Mod4/DIO2"=w961:bool, "Mod4/DIO3"=w960:bool)  [unwired: 2 in, 2 out]
    "Mod4/DIO2" <- w961
    "Mod4/DIO3" <- w960
    n324 = xnode "FPGA I/O Node"("error in"=w934) -> ("error out"=w951:errorcluster, "Mod5/DIO2"=w948:bool, "Mod5/DIO3"=w947:bool)  [unwired: 2 in, 2 out]
    "Mod5/DIO2" <- w948
    "Mod5/DIO3" <- w947
    n325 = xnode "FPGA I/O Node"("error in"=w934) -> ("error out"=w937:errorcluster, "Mod6/DIO0"=w943:bool, "Mod6/DIO1"=w942:bool)  [unwired: 2 in, 2 out]
    "Mod6/DIO0" <- w943
    "Mod6/DIO1" <- w942
    n326 = xnode "FPGA I/O Node"("error in"=w934) -> ("error out"=w952:errorcluster, "Mod5/DIO0"=w955:bool, "Mod5/DIO1"=w956:bool)  [unwired: 2 in, 2 out]
    "Mod5/DIO0" <- w955
    "Mod5/DIO1" <- w956
    n327 = xnode ("FPGA I/O Node")("error in"=w934) -> ("error out"=w962:errorcluster, "Mod4/DIO0"=w964:bool, "Mod4/DIO1"=w963:bool)  [unwired: 2 in, 2 out]
    "Mod4/DIO0" <- w964
    "Mod4/DIO1" <- w963
    n328 = xnode "FPGA I/O Node"("error in"=w934) -> ("error out"=w936:errorcluster, "Mod6/DIO2"=w938:bool, "Mod6/DIO3"=w939:bool)  [unwired: 2 in, 2 out]
    "Mod6/DIO2" <- w938
    "Mod6/DIO3" <- w939
    n329 = call "Tick Count"() -> ("Tick Count(Ticks)"=w979:u32)
    n330 = Subtract(x=w979, y=w978) -> (x-y=→"Measured Counter Time Period (Ticks)":u32)
    n331 = Merge Errors(w962, w957, w952, w951, w937, w936) -> (w935:errorcluster)
    "Interferometer Loop Error" <- w935
    n332 = call "Quadrature.vi"("Reset Counter"="Reset Optics X", "Quad A"=w964, "ticks in"=w977, "Last Quad B"=w965, "Last Quad A"=w966, "Quad B"=w963) -> ("ticks out"=w930:i32)  [unwired: 5 in]
    n333 = call "Quadrature.vi"("Reset Counter"="Reset Sample X", "Quad A"=w961, "ticks in"=w976, "Last Quad B"=w958, "Last Quad A"=w959, "Quad B"=w960) -> ("ticks out"=w931:i32)  [unwired: 5 in]
    n334 = call "Quadrature.vi"("Reset Counter"="Reset Optics Y", "Quad A"=w955, "ticks in"=w974, "Last Quad B"=w953, "Last Quad A"=w954, "Quad B"=w956) -> ("ticks out"=w932:i32)  [unwired: 5 in]
    n335 = call "Quadrature.vi"("Reset Counter"="Reset Sample Y", "Quad A"=w948, "ticks in"=w972, "Last Quad B"=w950, "Last Quad A"=w949, "Quad B"=w947) -> ("ticks out"=w929:i32)  [unwired: 5 in]
    n336 = call "Quadrature.vi"("Reset Counter"="Reset Optics Z", "Quad A"=w943, "ticks in"=w970, "Last Quad B"=w945, "Last Quad A"=w944, "Quad B"=w942) -> ("ticks out"=w928:i32)  [unwired: 5 in]
    n337 = call "Quadrature.vi"("Reset Counter"="Reset Sample Z", "Quad A"=w938, "ticks in"=w968, "Last Quad B"=w941, "Last Quad A"=w940, "Quad B"=w939) -> ("ticks out"=w927:i32)  [unwired: 5 in]
    n338 = xnode ("Register Write")("Data"=w932) -> ()  [unwired: 1 in, 1 out]
    n339 = xnode ("Register Write")("Data"=w930) -> ()  [unwired: 1 in, 1 out]
    n340 = xnode ("Register Write")("Data"=w931) -> ()  [unwired: 1 in, 1 out]
    n341 = xnode ("Register Write")("Data"=w929) -> ()  [unwired: 1 in, 1 out]
    n342 = Unbundle By Name(w935) -> ("status"=w933:bool)
    n343 = xnode ("Register Write")("Data"=w928) -> ()  [unwired: 1 in, 1 out]
    n344 = xnode ("Register Write")("Data"=w927) -> ()  [unwired: 1 in, 1 out]
    "Counter Loop iterations" <- w926
  }
  n345 = node-c288(w5) -> ()  [unwired: 1 out]
